vi "Do_ADAM_channel.vi"(3 "Current Time (sec)":dbl, 4 "Scan Period":dbl format="%.2f", 5 "Previous Scan Value":dbl format="%.2f", 6 "Present scan array":dbl[](array[numeric]) format="%.2f", 7 "Value to Output":dbl format="%.2f", 8 "Ch Description":T1 {"Duty" format="%016b"; "D" format="%#_5g"; "C" format="%#_5g"; "B" format="%#_5g"; "A" format="%#_5g"}, 9 "Ch names":string[](array[string])) -> (0 "Scan comment":string, 1 "Output":dbl format="%.3f", 2 "execTime":dbl caption="Execution Time" format="%_3ps")   [LabVIEW 2022 SP3]
uses:
  ADAM Client/Sub VIs/ADAM Controls/Ch_description_ADAM.ctl
  ADAM Client/Sub VIs/ADAM Controls/Module_type_ADAM.ctl
  ADAM Client/Sub VIs/ADAM Controls/Function_ADAM.ctl
  ADAM Client/Sub VIs/ADAM Controls/Channel_State.ctl
  ADAM Client/Sub VIs/ADAM Controls/Calib_type_ADAM.ctl
  ADAM Client/Sub VIs/ADAM Controls/Address.ctl
  ADAM Serial/Instrument drivers/TENMA 72-2xxx PSU/ctls/TENMA 72-2xxx commands.ctl
  ADAM Client/Sub VIs/ADAM Controls/Remember_value_mode.ctl
  ADAM Serial/Instrument drivers/Arduino/ctls_and_globals/Arduino tx msg cluster.ctl
  Anemometry/Anemometry Sub Vis/Controls/In_Range.ctl
  ADAM Client/Sub VIs/ADAM Controls/Update_scan_value.ctl
  Anemometry/Anemometry Sub Vis/Globals/Gas_management_global.vi
  ADAM_Global.vi
  Anemometry/Anemometry Sub Vis/Globals/EnFlo_Tunnel_Global.vi
  Anemometry/Anemometry Sub Vis/Globals/Constants_global.vi
  <vilib>/Analysis/NI_AALBase.lvlib
panel:
  in  "MaxAge(s)":dbl=1.5
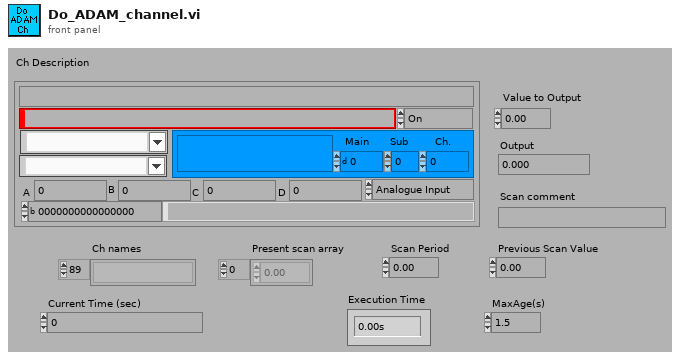
[diagram p1: front panel]
types:
  T1 = typedef "Ch_description_ADAM.ctl" = cluster{"Ch Name":string, "Type":T2, "Function":T3, "Ch State":T4, "Calibration type":T5, "A":dbl, "B":dbl, "C":dbl, "D":dbl, "Comments":string, "Address":T6, "String":string, "Duty":u16}
  T2 = typedef "Module_type_ADAM.ctl" = string
  T3 = typedef "Function_ADAM.ctl" = enum16{"Analogue Input", "Digital Input", "Event counter", "Event rate", "Analogue Output", "Digital Output", "Relay Output"}
  T4 = typedef "Channel_State.ctl" = enum16{"On", "Off", "Always On", "Always Off"}
  T5 = typedef "Calib_type_ADAM.ctl" = string
  T6 = typedef "Address.ctl" = cluster{"Main":i32, "Ch.":i32, "Sub":i32, "Port Name":string}
  T7 = typedef "TENMA 72-2xxx commands.ctl" = string
  T8 = typedef "Remember_value_mode.ctl" = enum16{"Read only", "Read and Write"}
  T9 = typedef "In_Range.ctl" = enum16{"%", "±", "% & ±"}
  T10 = enum16{"Append to Global", "Read Global then Clear"}
  T11 = typedef "Update_scan_value.ctl" = cluster{"Channel Name":string, "New Value":dbl, "!Auto_Off":bool}
  T12 = typedef "Arduino tx msg cluster.ctl" = cluster{"dest":u8, "A/D/C/I":string, "R/W":string, "chan":u8, "val (float)":sgl}
  T13 = typedef "Client_State_Cluster.ctl" = cluster{"Client Name":string, "Traverse level State":T14, "People to Email":string[], "Next Contact Time":dbl}
  T14 = typedef "Traverse_Level_State.ctl" = enum16{"Running", "Complete"}
  T15 = typedef "Modbus error cluster.ctl" = cluster{"Checksum ok":bool, "Modbus exception code":T16, "Response from correct drive":bool, "Comms error":errorcluster}
  T16 = typedef "Exception codes.ctl" = u8
  T17 = typedef "Extended drive status bits.ctl" = cluster{"Ready":bool, "Running":bool, "Tripped":bool, "Standby":bool, "Fire mode":bool, "Reserved (0)":bool, "Speed set-point reached":bool, "Below minimum speed":bool, "Overload":bool, "Mains loss":bool, "Heatsink >85°C":bool, "Control board >80°C":bool, "Switching frequency reduction":bool, "Reverse rotation":bool, "Reserved (0)":bool, "Live toggle bit":bool}
  T18 = typedef "Motor data.ctl" = cluster{"Motor RPM (/min)":dbl, "Motor current (A)":dbl, "Motor power (kW)":dbl, "Motor torque (%)":dbl}
  T19 = typedef "Further motor and drive data.ctl" = cluster{"Motor RMS voltage (V)":dbl, "Drive heatsink temperature (°C)":dbl, "Drive internal temperature (°C)":dbl, "Drive DC bus voltage (V)":dbl, "Drive fault code":T20}
  T20 = typedef "Drive fault codes.ctl" = u8
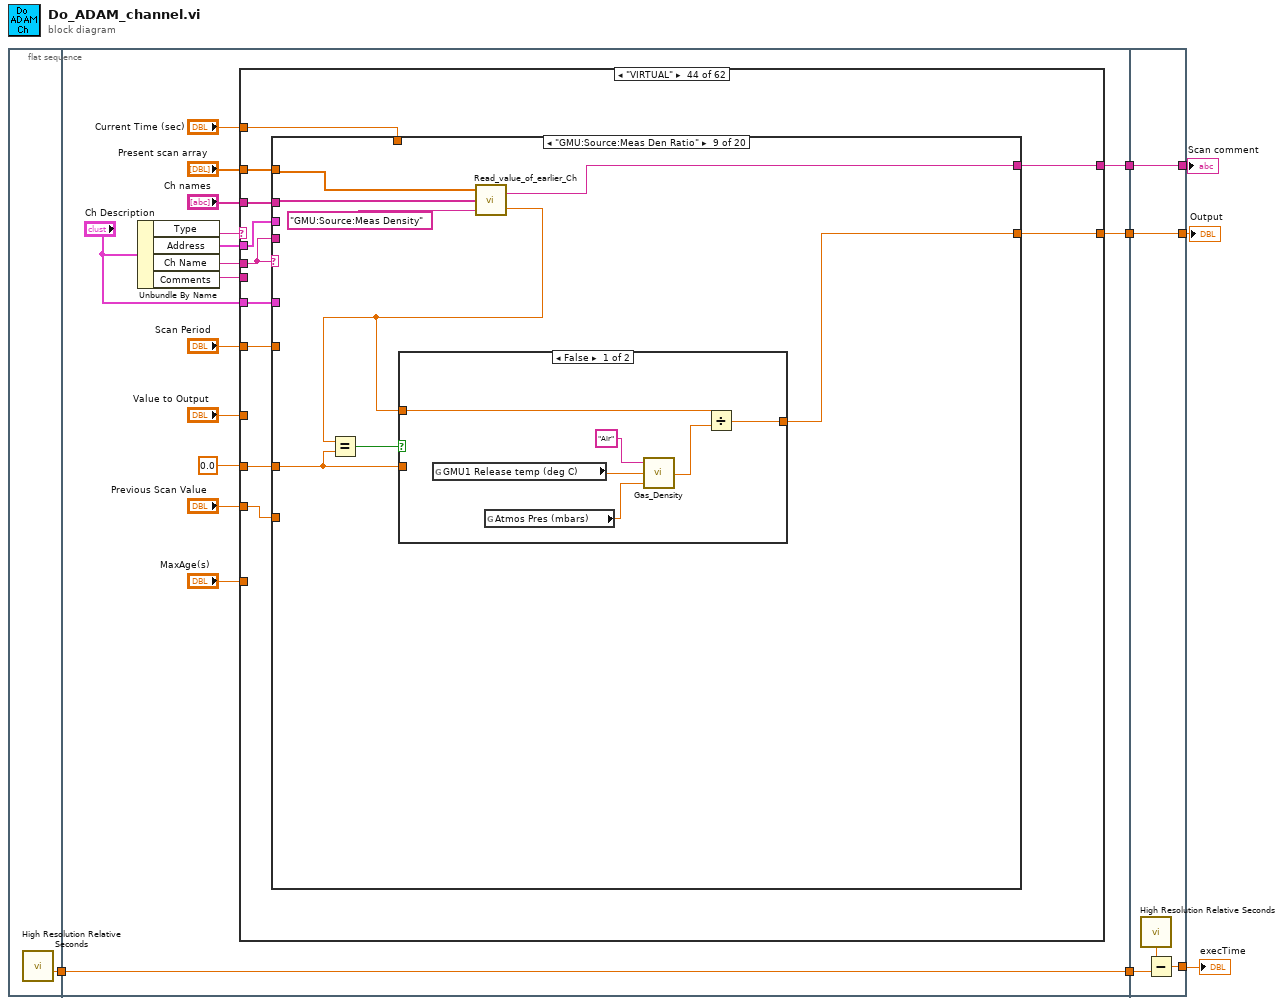
[diagram p0: block diagram]
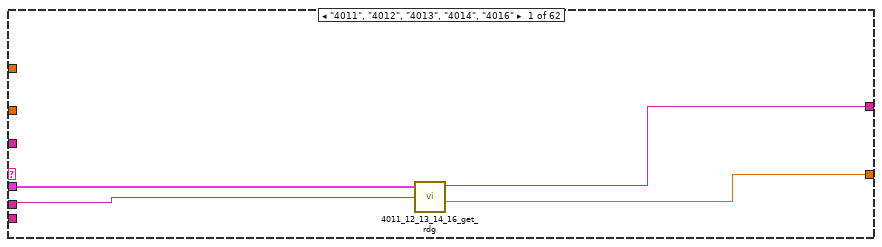
[diagram p2: hidden frame]
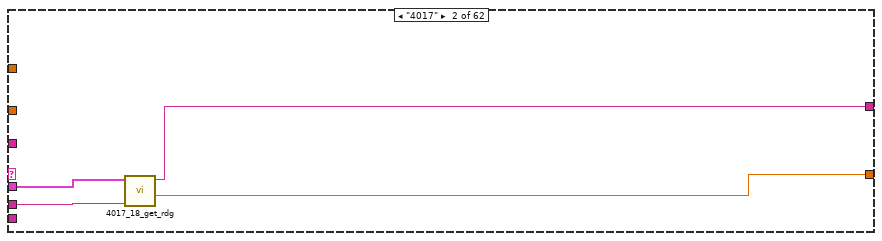
[diagram p3: hidden frame]
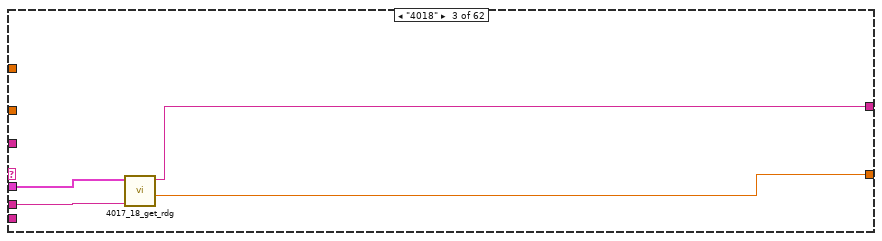
[diagram p4: hidden frame]
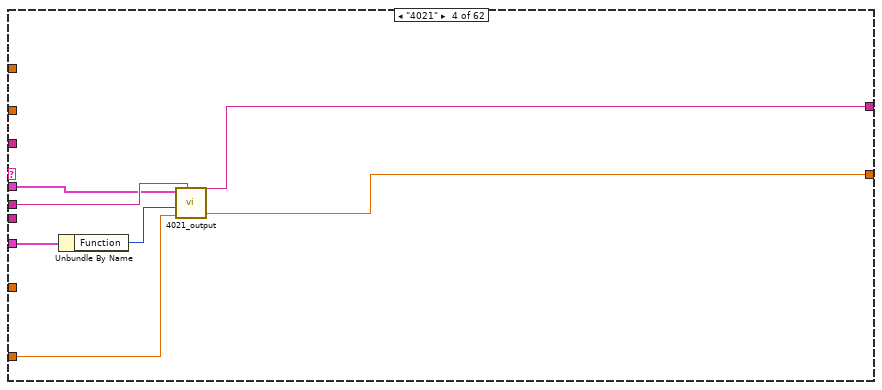
[diagram p5: hidden frame]
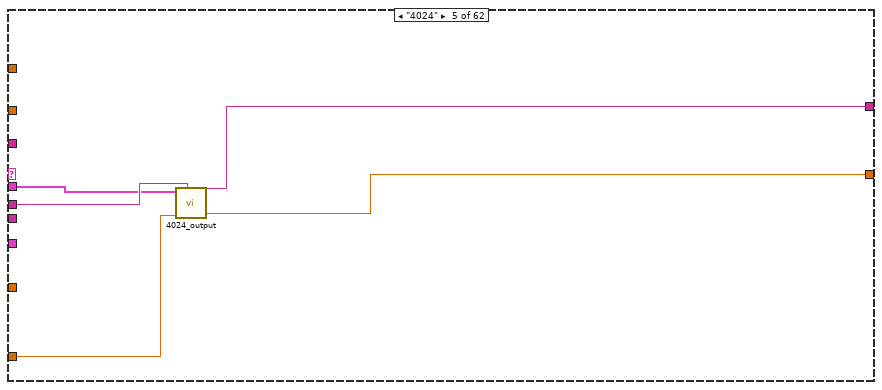
[diagram p6: hidden frame]
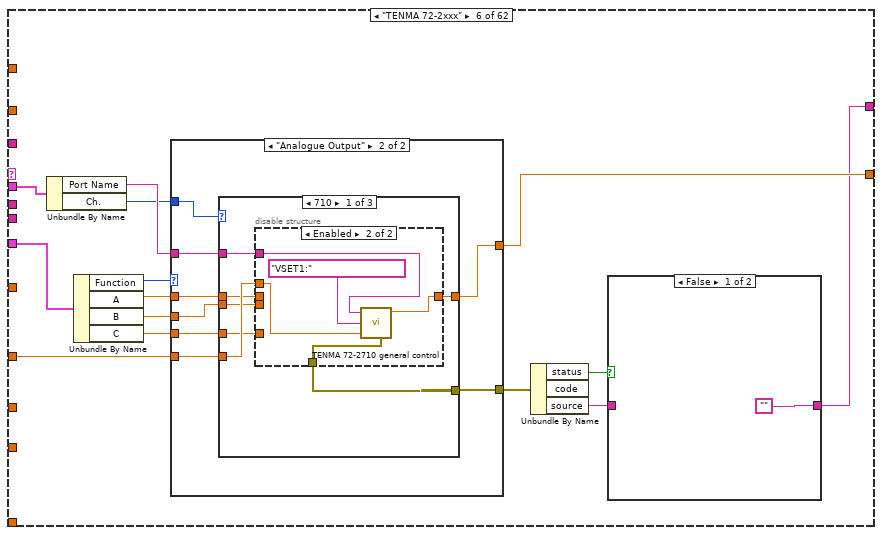
[diagram p7: hidden frame]
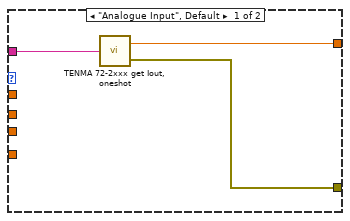
[diagram p8: hidden frame]
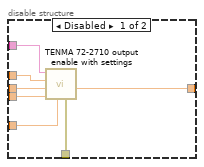
[diagram p9: hidden frame]
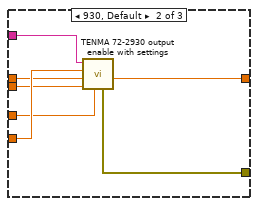
[diagram p10: hidden frame]
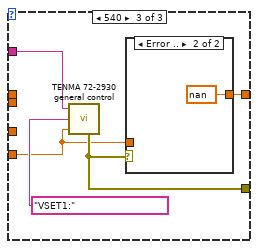
[diagram p11: hidden frame]
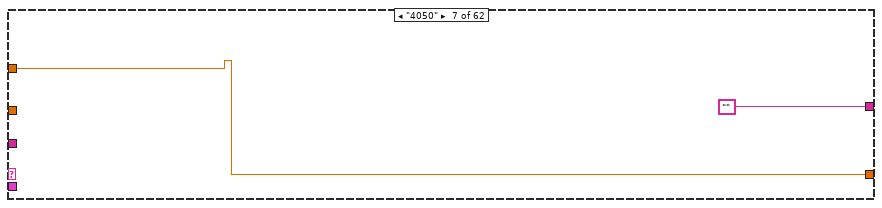
[diagram p14: hidden frame]
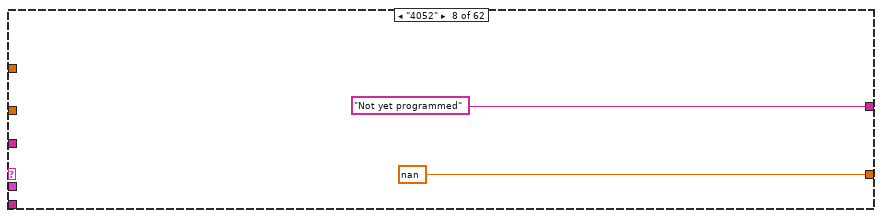
[diagram p15: hidden frame]
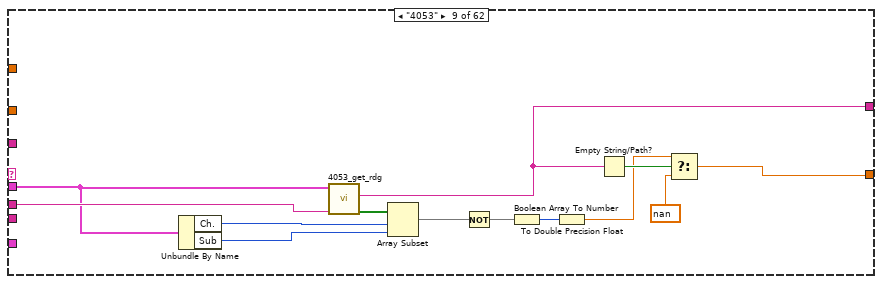
[diagram p16: hidden frame]
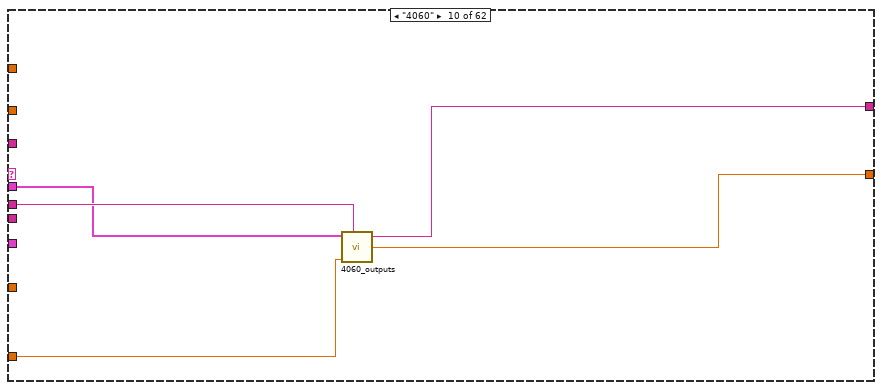
[diagram p17: hidden frame]
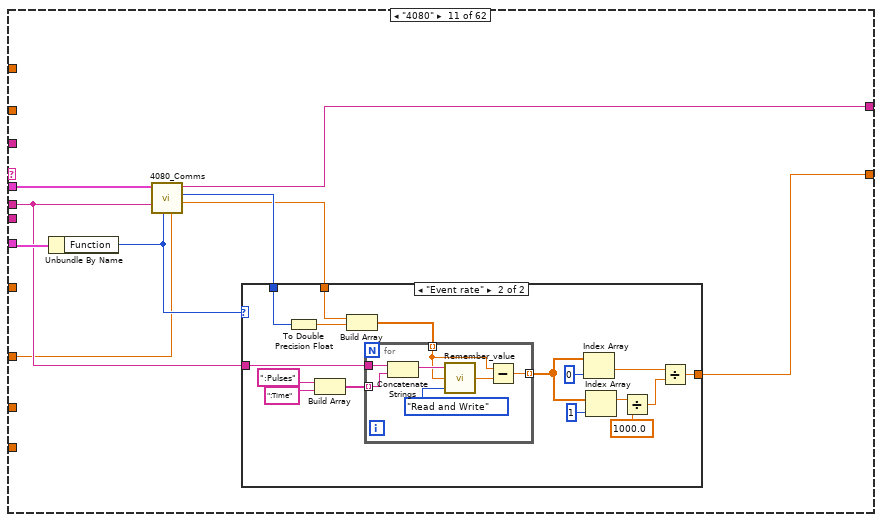
[diagram p18: hidden frame]
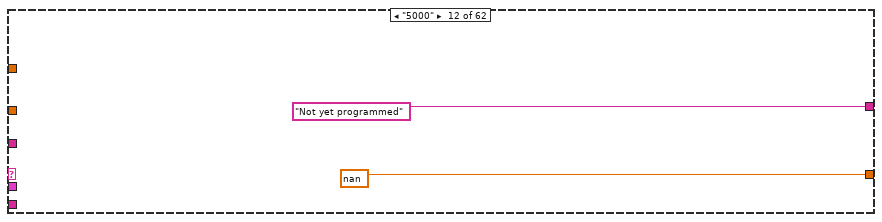
[diagram p20: hidden frame]
diagram:
  n1 = flat-sequence {
    tunnel: [w8] -> w3
    tunnel: [w11] -> w5
    tunnel: [w10] -> w4
    tunnel: w3 -> [w9]
    tunnel: [w9] -> w2
    tunnel: [w1603] -> w6
    tunnel: [w1604] -> w7
    tunnel: w5 -> [w1604]
    tunnel: w4 -> [w1603]
    tunnel: w2 -> [w1601]
    tunnel: [w1600] -> w1
    frame #0 {
      n2 = call <vilib>:"High Resolution Relative Seconds.vi"() -> ("relative seconds"=w8:dbl)
    }
    frame #1 {
      n3 = Unbundle By Name("Ch Description") -> ("Type"=w14:T2, "Address"=w22:T6, "Ch Name"=w16:string, "Comments"=w20:string)
      n4 = case shown="\"VIRTUAL\"" w14 {
        tunnel: [w27 w31 w35 w42 w47 w60 w109 nan w114 w128 w137 nan w167 w177 w209 w217 w238 w260 w280 w297 w313 w330 w360 w381 w486 w604 w606 nan w613 w615 w619 w626 w628 w644 w658 w662 w666 w673 w674 w680 w743 nan w752 w772 w1324 w1334 w1346 w1358 w1372 w1377 w1389 w1396 w1399 w1404 w1410 w1415 w1438 w1460 w1494 w1536 w1592 0.0 ("Output")] -> w10
        tunnel: [w28 w32 w36 w43 w48 w57 "" "Not yet programmed" w117 w129 w139 "Not yet programmed" w168 w180 w210 w216 w239 w261 w279 w296 w316 w332 w355 w380 w485 w605 w607 "Not yet programmed" w612 w616 w620 w625 w629 w643 w657 w663 w667 w672 w678 w682 w744 "Not yet programmed" "" w771 w1325 w1332 "" "" w1371 w1378 w1390 "" w1400 "" w1409 "" "Crazy time based random number!" w1449 w1495 w1537 w1591 "Warning; unmatched case in Do_ADAM_channel" ("Status note")] -> w11
        tunnel: w22 -> [w25 w29 w33 w37 w44 w61 _ _ w118 w127 w131 _ w169 w181 w211 w215 w240 w262 w294 w311 w328 w345 w371 w385 w490 w603 w608 _ _ _ _ w623 w627 w646 _ _ w669 w670 w676 w684 w749 _ w761 w763 _ _ _ _ _ _ _ _ _ _ _ _ _ _ w1499 w1538 _ _]
        tunnel: "Ch Description" -> [_ _ _ w41 _ w55 _ _ _ _ w138 _ _ w170 _ w214 w237 w259 _ _ _ _ _ _ _ _ _ _ w614 w618 w622 _ _ _ w659 w665 _ _ _ w683 _ _ _ w765 w1329 w1338 _ _ w1374 w1380 w1394 _ w1401 w1405 w1411 _ _ _ w1492 _ w1590 _]
        tunnel: w16 -> [w26 w30 w34 w38 w45 _ _ _ w125 w130 w134 _ w166 w176 w208 w212 w234 w256 w278 w295 w312 w329 w347 w377 w482 _ _ _ _ _ _ w624 _ w645 _ _ w668 w671 w677 w681 w748 _ _ w768 _ _ _ w1354 _ _ _ _ _ _ _ _ _ w1456 _ w1531 _ _]
        tunnel: "Ch names" -> [_ _ _ _ _ _ _ _ _ _ _ _ _ _ _ _ _ _ _ _ _ _ _ _ _ _ _ _ _ _ _ _ _ _ _ _ _ _ _ _ _ _ _ w770 w1330 w1337 _ _ w1375 w1381 w1395 _ w1402 _ _ _ _ _ _ _ w1597 _]
        tunnel: "Present scan array" -> [_ _ _ _ _ _ _ _ _ _ _ _ _ _ _ _ _ _ _ _ _ _ _ _ _ _ _ _ _ _ _ _ _ _ _ _ _ _ _ _ _ _ _ w769 w1328 w1335 _ _ w1373 w1379 w1393 _ w1403 _ _ _ _ _ _ _ w1595 _]
        tunnel: w20 -> [_ _ _ _ _ _ _ _ _ _ _ _ _ _ _ _ _ _ _ _ _ _ _ _ _ _ _ _ _ _ _ _ _ _ _ _ _ _ _ _ _ _ _ _ _ _ _ _ _ _ _ _ _ _ _ _ _ _ _ _ _ _]
        tunnel: "Value to Output" -> [_ _ _ w39 w46 w53 _ _ _ w126 w132 _ _ w172 _ w213 w235 w257 _ _ w314 w331 _ _ _ _ _ _ w611 w617 w621 _ _ w642 w660 w664 _ _ _ w679 _ _ w756 _ w1326 _ _ _ _ _ w1391 _ _ _ _ _ _ _ w1488 _ w1596 _]
        tunnel: "Scan Period" -> [_ _ _ _ _ _ _ _ _ _ _ _ _ _ _ _ _ _ _ _ _ _ _ _ _ _ _ _ _ _ _ _ _ _ _ _ _ _ _ _ _ _ _ w767 w1327 w1336 _ _ _ _ w1392 _ _ _ w1407 w1416 _ _ _ _ w1593 _]
        tunnel: "Previous Scan Value" -> [_ _ _ _ _ _ _ _ _ _ _ _ _ _ _ _ _ _ w282 w299 _ _ _ w379 w484 _ _ _ _ _ _ _ _ _ _ _ _ _ _ _ _ _ _ w766 w1323 _ w1346 _ w1370 w1376 w1388 w1396 _ _ w1408 w1413 _ _ _ _ w1594 _]
        tunnel: 0.0 -> [_ _ _ _ _ _ _ _ _ _ _ _ _ _ _ _ _ _ _ _ _ _ _ _ _ _ _ _ _ _ _ _ _ _ _ _ _ _ _ _ _ _ _ w764 _ _ _ _ _ _ _ _ _ _ _ _ _ _ _ _ _ _]
        tunnel: "MaxAge(s)" -> [_ _ _ _ _ _ _ _ _ _ _ _ _ _ _ _ _ _ _ _ _ _ _ _ _ _ _ _ _ _ _ _ _ _ w656 w661 _ _ _ _ _ _ _ _ _ _ _ _ _ _ _ _ _ _ _ _ _ _ _ _ _ _]
        tunnel: "Current Time (sec)" -> [_ _ _ _ _ _ w109 _ _ _ _ _ _ _ _ _ _ _ _ _ _ _ _ _ _ _ _ _ _ _ _ _ _ _ _ _ _ _ _ _ _ _ _ w762 _ _ _ _ _ _ _ _ _ _ _ _ w1431 w1439 _ _ _ _]
        frame "4011", "4012", "4013", "4014", "4016" {
          n5 = call "4011_12_13_14_16_get_rdg.vi"("Address"=w25, "Channel Name"=w26) -> ("Comment"=w28:string, "Reading"=w27:dbl)  [unwired: 1 in, 2 out]
        }
        frame "4017" {
          n6 = call "4017_18_get_rdg.vi"("Channel Name"=w30, "Address"=w29) -> ("Reading"=w31:dbl, "Comment"=w32:string)  [unwired: 2 in, 2 out]
        }
        frame "4018" {
          n7 = call "4017_18_get_rdg.vi"("Channel Name"=w34, "Address"=w33) -> ("Reading"=w35:dbl, "Comment"=w36:string)  [unwired: 2 in, 2 out]
        }
        frame "4021" {
          n8 = Unbundle By Name(w41) -> ("Function"=w40:T3)
          n9 = call "4021_output.vi"("Address"=w37, "Function"=w40, "Set to:"=w39, "Channel Name"=w38) -> ("Comment"=w43:string, "Reading"=w42:dbl)  [unwired: 1 in, 1 out]
        }
        frame "4024" {
          n10 = call "4024_output.vi"("Address"=w44, "Set to:"=w46, "Channel Name"=w45) -> ("Comment"=w48:string, "Reading"=w47:dbl)  [unwired: 3 in]
        }
        frame "TENMA 72-2xxx" {
          n11 = Unbundle By Name(w61) -> ("Port Name"=w62:string, "Ch."=w49:i32)
          n12 = Unbundle By Name(w55) -> ("Function"=w54:T3, "A"=w52:dbl, "B"=w51:dbl, "C"=w50:dbl)
          n13 = case shown="\"Analogue Output\"" w54 {
            tunnel: w62 -> [w65 w73]
            tunnel: [w64 w67] -> w60
            tunnel: [w63 w68] -> w59
            tunnel: w53 -> [_ w72]
            tunnel: w52 -> [_ w71]
            tunnel: w51 -> [_ w70]
            tunnel: w50 -> [_ w69]
            tunnel: w49 -> [_ w66]
            frame "Analogue Input", Default {
              n14 = call "TENMA 72-2xxx get Iout, oneshot.vi"("Port"=w65) -> ("Iout (A)"=w64:sgl, "error out"=w63:errorcluster)
            }
            frame "Analogue Output" {
              n15 = case shown="710" w66 {
                tunnel: w73 -> [w80 w99 w104]
                tunnel: w72 -> [w79 w98 w100]
                tunnel: w71 -> [w78 w97 _]
                tunnel: w70 -> [w77 w96 _]
                tunnel: w69 -> [w76 w95 _]
                tunnel: [w75 w94 w102] -> w68
                tunnel: [w74 w93 w101] -> w67
                frame 710 {
                  n16 = disable-structure shown="Enabled" {
                    disable-tunnel: w80 -> [w87 w91]
                    disable-tunnel: w79 -> [w86 w88]
                    disable-tunnel: w78 -> [w85 _]
                    disable-tunnel: w77 -> [w84 _]
                    disable-tunnel: w76 -> [w83 _]
                    disable-tunnel: [w82 w89] -> w75
                    disable-tunnel: [w81 w90] -> w74
                    frame Disabled {
                      n17 = call "TENMA 72-2710 output enable with settings.vi"("Initial wait (ms)"=w83, "Running current limit (A)"=w84, "Initial current limit (A)"=w85, "Voltate output (V)"=w86, "Port"=w87) -> ("Returned voltage output (V)"=w81:sgl, "Error out"=w82:errorcluster)  [unwired: 2 in, 3 out]
                    }
                    frame Enabled {
                      n18 = call "TENMA 72-2710 general control.vi"("Value to set"=w88, "Command"=T7 "VSET1:", "Port"=w91) -> ("error out"=w89:errorcluster, "Returned value"=w90:sgl)  [unwired: 1 in, 3 out]
                    }
                  }
                }
                frame 930, Default {
                  n19 = call "TENMA 72-2930 output enable with settings.vi"("Initial wait (ms)"=w95, "Running current limit (A)"=w96, "Initial current limit (A)"=w97, "Voltate output (V)"=w98, "Port"=w99) -> ("Returned voltage output (V)"=w93:sgl, "Error out"=w94:errorcluster)  [unwired: 2 in, 3 out]
                }
                frame 540 {
                  n20 = call "TENMA 72-2930 general control.vi"("Value to set"=w100, "Command"=T7 "VSET1:", "Port"=w104) -> ("error out"=w102:errorcluster)  [unwired: 1 in, 4 out]
                  n21 = case shown="Error .." w102 {
                    tunnel: [w105 nan ("Value to Output")] -> w101
                    tunnel: w100 -> [w105 _]
                    frame No Error {
                    }
                    frame Error {
                    }
                  }
                }
              }
            }
          }
          n22 = Unbundle By Name(w59) -> ("status"=w58:bool, "source"=w56:string)  [unwired: 1 out]
          n23 = case shown="False" w58 {
            tunnel: ["" w108] -> w57
            tunnel: w56 -> [_ w108]
            frame False {
            }
            frame True {
            }
          }
        }
        frame "4050" {
        }
        frame "4052" {
        }
        frame "4053" {
          n24 = Unbundle By Name(w118) -> ("Ch."=w119:i32, "Sub"=w124:i32)
          n25 = call "4053_get_rdg.vi"("Channel Name"=w125, "Address"=w118) -> ("Boolean array"=w123:bool[], "Comment"=w117:string)  [unwired: 2 in, 2 out]
          n26 = Array Subset(array=w123, index=w119, length=w124) -> (w122:bool[])
          n27 = Not(x=w122) -> (.not. x?=w120:bool[])
          n28 = Boolean Array To Number(Boolean array=w120) -> (number=w121:u32)
          n29 = To Double Precision Float(number=w121) -> (double precision float=w115:dbl)
          n30 = Empty String/Path?(string/path=w117) -> (empty?=w116:bool)
          n31 = Select(t=w115, s=w116, f=nan) -> (s? t:f=w114:dbl)
        }
        frame "4060" {
          n32 = call "4060_outputs.vi"("Address"=w127, "Value to Output"=w126, "Channel Name"=w130) -> ("Comment"=w129:string, "Reading"=w128:dbl)  [unwired: 2 in, 1 out]
        }
        frame "4080" {
          n33 = Unbundle By Name(w138) -> ("Function"=w133:T3)
          n34 = call "4080_Comms.vi"("Value to display"=w132, "Function"=w133, "Channel Name"=w134, "Address"=w131) -> ("Reading"=w135:dbl, "millisecond timer value"=w136:u32, "Comment"=w139:string)  [unwired: 2 in, 1 out]
          n35 = case shown="\"Event rate\"" w133 {
            tunnel: w134 -> [_ w156]
            tunnel: w136 -> [_ w149]
            tunnel: [w140 w141] -> w137
            tunnel: w135 -> [w140 w150]
            frame "Event counter", Default {
            }
            frame "Event rate" {
              n36 = To Double Precision Float(number=w149) -> (double precision float=w148:dbl)
              n37 = Build Array(":Pulses", ":Time") -> (w151:string[])
              n38 = Build Array(w150, w148) -> (w147:dbl[])
              n39 = for {
                tunnel: w156 -> [w160]
                tunnel: [w161] -> w144 mode=indexing
                tunnel: w151 -> [w158] mode=indexing
                tunnel: w147 -> [w157] mode=indexing
                n40 = Concatenate Strings(w160, w158) -> (w159:string)
                n41 = call "Remember_value.vi"("Mode"=Remember_value_mode."Read and Write", "Input Value"=w157, "Ch name"=w159) -> ("Output Value"=w162:dbl)
                n42 = Subtract(x=w157, y=w162) -> (x-y=w161:dbl)
              }
              n43 = Index Array(array=w144, index=0) -> (element=w142:dbl)
              n44 = Index Array(array=w144, index=1) -> (element=w143:dbl)
              n45 = Divide(x=w143, y=1000.0) -> (x/y=w154:dbl)
              n46 = Divide(x=w142, y=w154) -> (x/y=w141:dbl)
            }
          }
        }
        frame "5000" {
        }
        frame "5017", "5018" {
          n47 = call "5017_18_get_rdg.vi"("Address (all reqd.)"=w169, "Channel Name"=w166) -> ("Comment"=w168:string, "Reading"=w167:dbl)  [unwired: 3 out]
        }
        frame "5024" {
          n48 = Less Than 0?(x=w172) -> (x < 0?=w175:bool)
          n49 = Unbundle By Name(w170) -> ("Calibration type"=w171:T5)
          n50 = case shown="False" w175 {
            tunnel: [w187 0.0 ("t")] -> w173
            tunnel: w172 -> [w185 _]
            tunnel: w171 -> [w186 _]
            tunnel: w170 -> [w184 _]
            frame False {
              n51 = case shown="\"Dx^3 + Cx^2 + Bx + A\"" w186 {
                tunnel: w185 -> [w188 w191 w197 w203]
                tunnel: w184 -> [_ w194 w200 w206]
                tunnel: [w188 w189 w195 w201] -> w187
                frame "Raw", Default {
                }
                frame "Bx + A" {
                  n52 = Unbundle By Name(w194) -> ("A"=w193:dbl)
                  n53 = Equal?(x=w193, y=w191) -> (x = y?=w192:bool)
                  n54 = Select(t=0.0, s=w192, f=w191) -> (s? t:f=w189:dbl)
                }
                frame "Cx^2 + Bx + A" {
                  n55 = Unbundle By Name(w200) -> ("A"=w199:dbl)
                  n56 = Equal?(x=w199, y=w197) -> (x = y?=w198:bool)
                  n57 = Select(t=0.0, s=w198, f=w197) -> (s? t:f=w195:dbl)
                }
                frame "Dx^3 + Cx^2 + Bx + A" {
                  n58 = Unbundle By Name(w206) -> ("A"=w205:dbl)
                  n59 = Equal?(x=w205, y=w203) -> (x = y?=w204:bool)
                  n60 = Select(t=0.0, s=w204, f=w203) -> (s? t:f=w201:dbl)
                }
              }
            }
            frame True {
            }
          }
          n61 = call "5024_set_output.vi"("Set to:"=w173, "Address (all reqd.)"=w181, "Channel Name"=w176) -> ("Comment"=w180:string, "Good Reply"=w178:bool)  [unwired: 2 out]
          n62 = case shown="\"Bx + A\", Default" w171 {
            tunnel: [w182 w183] -> w174
            tunnel: w173 -> [w182 _]
            tunnel: w172 -> [_ w183]
            frame "Raw" {
            }
            frame "Bx + A", Default {
            }
          }
          n63 = Select(t=w174, s=w178, f=nan) -> (s? t:f=w177:dbl)
        }
        frame "5051" {
          n64 = call "5051_56_get_inputs.vi"("Address (Main, Sub reqd.)"=w211, "Channel Name"=w208) -> ("Comment"=w210:string, "Single output"=w209:dbl)  [unwired: 3 out]
        }
        frame "5056" {
          n65 = Unbundle By Name(w214) -> ("Function"=w218:T3)
          n66 = case shown="\"Relay Output\"" w218 {
            tunnel: w215 -> [_ w224 w233]
            tunnel: ["This function is not available" w225 w231] -> w216
            tunnel: [nan ("A") w222 w228] -> w217
            tunnel: w213 -> [_ _ w227]
            tunnel: w212 -> [_ w221 w226]
            frame "Analogue Input", Default {
            }
            frame "Digital Input" {
              # "Readback value"
              n67 = call "5060_check_outputs.vi"("Address (Main, Sub reqd.)"=w224, "Channel Name"=w221) -> ("Comment"=w225:string, "Single Channel"=w223:i16)  [unwired: 3 out]
              n68 = To Double Precision Float(number=w223) -> (double precision float=w222:dbl)
            }
            frame "Relay Output" {
              # "Sets single o/p channel"
              n69 = Greater Than 0?(x=w227) -> (x > 0?=w232:bool)
              n70 = call "5056_60_set_single_output.vi"("Channel Name"=w226, "Address (all reqd.)"=w233, "Set state:"=w232) -> ("Comment"=w231:string, "Good Reply"=w230:bool)  [unwired: 2 out]
              n71 = Select(t=w227, s=w230, f=nan) -> (s? t:f=w228:dbl)
            }
          }
        }
        frame "5060" {
          n72 = Unbundle By Name(w237) -> ("Function"=w236:T3)
          n73 = case shown="\"Relay Output\"" w236 {
            tunnel: w240 -> [_ w246 w255]
            tunnel: ["This function is not available" w247 w253] -> w239
            tunnel: [nan ("A") w244 w250] -> w238
            tunnel: w235 -> [_ _ w249]
            tunnel: w234 -> [_ w243 w248]
            frame "Analogue Input", Default {
            }
            frame "Digital Input" {
              # "Readback value"
              n74 = call "5060_check_outputs.vi"("Address (Main, Sub reqd.)"=w246, "Channel Name"=w243) -> ("Comment"=w247:string, "Single Channel"=w245:i16)  [unwired: 3 out]
              n75 = To Double Precision Float(number=w245) -> (double precision float=w244:dbl)
            }
            frame "Relay Output" {
              # "Sets single o/p channel"
              n76 = Greater Than 0?(x=w249) -> (x > 0?=w254:bool)
              n77 = call "5056_60_set_single_output.vi"("Channel Name"=w248, "Address (all reqd.)"=w255, "Set state:"=w254) -> ("Comment"=w253:string, "Good Reply"=w252:bool)  [unwired: 2 out]
              n78 = Select(t=w249, s=w252, f=nan) -> (s? t:f=w250:dbl)
            }
          }
        }
        frame "6060" {
          n79 = Unbundle By Name(w259) -> ("Function"=w258:T3)
          n80 = case shown="\"Relay Output\"" w258 {
            tunnel: w262 -> [_ w268 w277]
            tunnel: ["This function is not available" w269 w275] -> w261
            tunnel: [nan ("A") w266 w272] -> w260
            tunnel: w257 -> [_ _ w271]
            tunnel: w256 -> [_ w265 w270]
            frame "Analogue Input", Default {
            }
            frame "Digital Input" {
              n81 = call "6060_read_all_I-O.vi"("Address (Main, Sub reqd.)"=w268, "Channel Name"=w265) -> ("Comment"=w269:string, "Single Input Channel"=w267:i16)  [unwired: 3 out]
              n82 = To Double Precision Float(number=w267) -> (double precision float=w266:dbl)
            }
            frame "Relay Output" {
              # "Sets single o/p channel"
              n83 = Greater Than 0?(x=w271) -> (x > 0?=w276:bool)
              n84 = call "6060_set_single_output.vi"("Channel Name"=w270, "Address (Main, Ch requd.)"=w277, "Set state:"=w276) -> ("Comment"=w275:string, "Good Reply"=w274:bool)  [unwired: 2 out]
              n85 = Select(t=w271, s=w274, f=nan) -> (s? t:f=w272:dbl)
            }
          }
        }
        frame "Arduino A_in" {
          w288 = T12 {"dest"=1, "A/D/C/I"="A", "R/W"="R", "chan"=1, "val (float)"=0.0}  # Tx msg cluster
          # "Analogue read case"
          n86 = Unbundle By Name(w294) -> ("Port Name"=w285:string, "Main"=w286:i32, "Ch."=w287:i32)
          n87 = To Unsigned Byte Integer(number=w286) -> (unsigned 8bit integer=w293:u8)
          n88 = To Unsigned Byte Integer(number=w287) -> (unsigned 8bit integer=w291:u8)
          n89 = Bundle By Name(cluster=w288, "dest"=w293, "A/D/C/I"="A" ("A/D"), "R/W"="R", "chan"=w291, "val (float)"=sgl 0.0) -> (w284:T12)
          n90 = call "Arduino generic wrapper.vi"("Tx msg cluster"=w284, "Channel Name"=w278, "Port name"=w285) -> ("Scan comment"=w279:string, "Output"=w281:dbl)
          n91 = Empty String/Path?(string/path=w279) -> (empty?=w283:bool)
          n92 = Select(t=w281, s=w283, f=w282) -> (s? t:f=w280:dbl)
        }
        frame "Pref" {
          w305 = T12 {"dest"=1, "A/D/C/I"="A", "R/W"="R", "chan"=1, "val (float)"=0.0}  # Tx msg cluster
          # "Analogue read case"
          n93 = Unbundle By Name(w311) -> ("Port Name"=w302:string, "Main"=w303:i32, "Ch."=w304:i32)
          n94 = To Unsigned Byte Integer(number=w303) -> (unsigned 8bit integer=w310:u8)
          n95 = To Unsigned Byte Integer(number=w304) -> (unsigned 8bit integer=w308:u8)
          n96 = Bundle By Name(cluster=w305, "dest"=w310, "A/D/C/I"="P" ("A/D"), "R/W"="R", "chan"=w308, "val (float)"=sgl 0.0) -> (w301:T12)
          n97 = call "Arduino generic wrapper.vi"("Tx msg cluster"=w301, "Channel Name"=w295, "Port name"=w302) -> ("Scan comment"=w296:string, "Output"=w298:dbl)
          n98 = Empty String/Path?(string/path=w296) -> (empty?=w300:bool)
          n99 = Select(t=w298, s=w300, f=w299) -> (s? t:f=w297:dbl)
        }
        frame "Arduino A_out" {
          w323 = T12 {"dest"=1, "A/D/C/I"="A", "R/W"="R", "chan"=1, "val (float)"=0.0}  # Tx msg cluster
          # "Analogue write case"
          n100 = Unbundle By Name(w328) -> ("Port Name"=w320:string, "Main"=w321:i32, "Ch."=w322:i32)
          n101 = To Unsigned Byte Integer(number=w321) -> (unsigned 8bit integer=w327:u8)
          n102 = To Unsigned Byte Integer(number=w322) -> (unsigned 8bit integer=w326:u8)
          n103 = To Single Precision Float(number=w314) -> (single precision float=w318:sgl)
          n104 = Bundle By Name(cluster=w323, "dest"=w327, "A/D/C/I"="A" ("A/D"), "R/W"="W", "chan"=w326, "val (float)"=w318) -> (w319:T12)
          n105 = call "Arduino generic wrapper.vi"("Tx msg cluster"=w319, "Channel Name"=w312, "Port name"=w320) -> ("Scan comment"=w316:string)  [unwired: 1 out]
          n106 = Empty String/Path?(string/path=w316) -> (empty?=w315:bool)
          n107 = Select(t=w314, s=w315, f=nan ("Reading")) -> (s? t:f=w313:dbl)
        }
        frame "Arduino D_out" {
          w340 = T12 {"dest"=1, "A/D/C/I"="A", "R/W"="R", "chan"=1, "val (float)"=0.0}  # Tx msg cluster
          # "Digital write case"
          n108 = Unbundle By Name(w345) -> ("Port Name"=w337:string, "Main"=w338:i32, "Ch."=w339:i32)
          n109 = To Unsigned Byte Integer(number=w338) -> (unsigned 8bit integer=w344:u8)
          n110 = To Unsigned Byte Integer(number=w339) -> (unsigned 8bit integer=w343:u8)
          n111 = To Single Precision Float(number=w331) -> (single precision float=w335:sgl)
          n112 = Bundle By Name(cluster=w340, "dest"=w344, "A/D/C/I"="D" ("A/D"), "R/W"="W", "chan"=w343, "val (float)"=w335) -> (w336:T12)
          n113 = call "Arduino generic wrapper.vi"("Tx msg cluster"=w336, "Channel Name"=w329, "Port name"=w337) -> ("Scan comment"=w332:string)  [unwired: 1 out]
          n114 = Empty String/Path?(string/path=w332) -> (empty?=w333:bool)
          n115 = Select(t=w331, s=w333, f=nan ("Reading")) -> (s? t:f=w330:dbl)
        }
        frame "Arduino Thermistor" {
          w365 = T12 {"dest"=1, "A/D/C/I"="A", "R/W"="R", "chan"=1, "val (float)"=0.0}  # Tx msg cluster
          # "Thermistor read case"
          # "values not expected in 'normal' operating conditions"
          n116 = Unbundle By Name(w371) -> ("Port Name"=w362:string, "Main"=w363:i32, "Ch."=w364:i32)
          n117 = To Unsigned Byte Integer(number=w363) -> (unsigned 8bit integer=w370:u8)
          n118 = To Unsigned Byte Integer(number=w364) -> (unsigned 8bit integer=w368:u8)
          n119 = Bundle By Name(cluster=w365, "dest"=w370, "A/D/C/I"="A" ("A/D"), "R/W"="R", "chan"=w368, "val (float)"=sgl 0.0) -> (w361:T12)
          n120 = call "Arduino generic wrapper.vi"("Tx msg cluster"=w361, "Channel Name"=w347, "Port name"=w362) -> ("Scan comment"=w351:string, "Output"=w349:dbl)
          n121 = Empty String/Path?(string/path=w351) -> (empty?=w350:bool)
          n122 = Select(t=w349, s=w350, f=nan) -> (s? t:f=w348:dbl)
          n123 = Less?(x=w349, y=-40.0) -> (x < y?=w352:bool)
          n124 = Greater?(x=w349, y=140.0) -> (0:w353:bool)
          n125 = case shown="False" w352 {
            tunnel: [w373 "Faulty thermistor open-circuit;"] -> w354
            tunnel: w353 -> [w372 _]
            frame False {
              n126 = case shown="False" w372 {
                tunnel: ["" "Faulty thermistor short-circuit;"] -> w373
                frame False {
                }
                frame True {
                }
              }
            }
            frame True {
            }
          }
          n127 = Or(x=w352, y=w353) -> (x .or. y?=w357:bool)
          n128 = Select(t=nan ("f"), s=w357, f=w348) -> (s? t:f=w360:dbl)
          n129 = Concatenate Strings(w351, w354) -> (w355:string)
        }
        frame "NaMCU" {
          # "See \"Default\" tab for channel matrix"
          # "PN's \"NaMCU\" devices. Low range pressure transducer with on-board correction, environmental sensor, 2x thermistors, Ain + Aout (5V), Din + Dout"
          n130 = Unbundle By Name(w385) -> ("Port Name"=w382:string, "Main"=w383:i32, "Sub"=w378:i32, "Ch."=w384:i32)
          n131 = case shown="4" w378 {
            tunnel: w384 -> [w395 w420 w441 w457 w473 _]
            tunnel: w383 -> [w394 w419 w440 w456 w472 _]
            tunnel: w382 -> [w393 w418 w439 w455 w471 _]
            tunnel: [w387 w416 w433 w449 w465 0.0 ("Output")] -> w381
            tunnel: [w388 w411 w435 w451 w467 "Warning; invalid Sub being addressed on a NaMCU device in Do_ADAM_channel.vi"] -> w380
            tunnel: w379 -> [w389 w403 w436 w452 w468 _]
            tunnel: w377 -> [w386 w402 w432 w448 w464 _]
            frame 0 {
              w396 = T12 {"dest"=1, "A/D/C/I"="A", "R/W"="R", "chan"=1, "val (float)"=0.0}  # Tx msg cluster
              # "Get pressure (Pa)"
              n132 = To Unsigned Byte Integer(number=w394) -> (unsigned 8bit integer=w401:u8)
              n133 = To Unsigned Byte Integer(number=w395) -> (unsigned 8bit integer=w399:u8)
              n134 = Bundle By Name(cluster=w396, "dest"=w401, "A/D/C/I"="P" ("A/D"), "R/W"="R", "chan"=w399, "val (float)"=sgl 0.0) -> (w392:T12)
              n135 = call "Arduino generic wrapper.vi"("Tx msg cluster"=w392, "Channel Name"=w386, "Port name"=w393) -> ("Scan comment"=w388:string, "Output"=w390:dbl)
              n136 = Empty String/Path?(string/path=w388) -> (empty?=w391:bool)
              n137 = Select(t=w390, s=w391, f=w389) -> (s? t:f=w387:dbl)
            }
            frame 1 {
              w421 = T12 {"dest"=1, "A/D/C/I"="A", "R/W"="R", "chan"=1, "val (float)"=0.0}  # Tx msg cluster
              # "values not expected in 'normal' operating conditions"
              # "Get temperature (deg C)"
              n138 = To Unsigned Byte Integer(number=w419) -> (unsigned 8bit integer=w426:u8)
              n139 = To Unsigned Byte Integer(number=w420) -> (unsigned 8bit integer=w424:u8)
              n140 = Bundle By Name(cluster=w421, "dest"=w426, "A/D/C/I"="T" ("A/D"), "R/W"="R", "chan"=w424, "val (float)"=sgl 0.0) -> (w417:T12)
              n141 = call "Arduino generic wrapper.vi"("Tx msg cluster"=w417, "Channel Name"=w402, "Port name"=w418) -> ("Scan comment"=w407:string, "Output"=w405:dbl)
              n142 = Empty String/Path?(string/path=w407) -> (empty?=w406:bool)
              n143 = Select(t=w405, s=w406, f=w403) -> (s? t:f=w404:dbl)
              n144 = Less?(x=w405, y=-40.0) -> (x < y?=w408:bool)
              n145 = Greater?(x=w405, y=140.0) -> (0:w409:bool)
              n146 = case shown="False" w408 {
                tunnel: [w428 "Faulty thermistor open-circuit;"] -> w410
                tunnel: w409 -> [w427 _]
                frame False {
                  n147 = case shown="True" w427 {
                    tunnel: ["" "Faulty thermistor short-circuit;"] -> w428
                    frame False {
                    }
                    frame True {
                    }
                  }
                }
                frame True {
                }
              }
              n148 = Or(x=w408, y=w409) -> (x .or. y?=w413:bool)
              n149 = Select(t=nan ("f"), s=w413, f=w404) -> (s? t:f=w416:dbl)
              n150 = Concatenate Strings(w407, w410) -> (w411:string)
            }
            frame 2 {
              w442 = T12 {"dest"=1, "A/D/C/I"="A", "R/W"="R", "chan"=1, "val (float)"=0.0}  # Tx msg cluster
              # "Get relative humidity (%)"
              n151 = To Unsigned Byte Integer(number=w440) -> (unsigned 8bit integer=w447:u8)
              n152 = To Unsigned Byte Integer(number=w441) -> (unsigned 8bit integer=w445:u8)
              n153 = Bundle By Name(cluster=w442, "dest"=w447, "A/D/C/I"="H" ("A/D"), "R/W"="R", "chan"=w445, "val (float)"=sgl 0.0) -> (w438:T12)
              n154 = call "Arduino generic wrapper.vi"("Tx msg cluster"=w438, "Channel Name"=w432, "Port name"=w439) -> ("Scan comment"=w435:string, "Output"=w434:dbl)
              n155 = Empty String/Path?(string/path=w435) -> (empty?=w437:bool)
              n156 = Select(t=w434, s=w437, f=w436) -> (s? t:f=w433:dbl)
            }
            frame 3 {
              w458 = T12 {"dest"=1, "A/D/C/I"="A", "R/W"="R", "chan"=1, "val (float)"=0.0}  # Tx msg cluster
              # "Get fluid density (kg/m^3)"
              n157 = To Unsigned Byte Integer(number=w456) -> (unsigned 8bit integer=w463:u8)
              n158 = To Unsigned Byte Integer(number=w457) -> (unsigned 8bit integer=w461:u8)
              n159 = Bundle By Name(cluster=w458, "dest"=w463, "A/D/C/I"="R" ("A/D"), "R/W"="R", "chan"=w461, "val (float)"=sgl 0.0) -> (w454:T12)
              n160 = call "Arduino generic wrapper.vi"("Tx msg cluster"=w454, "Channel Name"=w448, "Port name"=w455) -> ("Scan comment"=w451:string, "Output"=w450:dbl)
              n161 = Empty String/Path?(string/path=w451) -> (empty?=w453:bool)
              n162 = Select(t=w450, s=w453, f=w452) -> (s? t:f=w449:dbl)
            }
            frame 4 {
              w474 = T12 {"dest"=1, "A/D/C/I"="A", "R/W"="R", "chan"=1, "val (float)"=0.0}  # Tx msg cluster
              # "Get flow speed (pitot-static equivalent) (m/s)"
              n163 = To Unsigned Byte Integer(number=w472) -> (unsigned 8bit integer=w479:u8)
              n164 = To Unsigned Byte Integer(number=w473) -> (unsigned 8bit integer=w477:u8)
              n165 = Bundle By Name(cluster=w474, "dest"=w479, "A/D/C/I"="U" ("A/D"), "R/W"="R", "chan"=w477, "val (float)"=sgl 0.0) -> (w470:T12)
              n166 = call "Arduino generic wrapper.vi"("Tx msg cluster"=w470, "Channel Name"=w464, "Port name"=w471) -> ("Scan comment"=w467:string, "Output"=w466:dbl)
              n167 = Empty String/Path?(string/path=w467) -> (empty?=w469:bool)
              n168 = Select(t=w466, s=w469, f=w468) -> (s? t:f=w465:dbl)
            }
            frame Default {
              # "dP_sensor and flow speed are time-averaged between calls"
              # "Oh dear, user has created a server channel with an invalid \"sub\" address"
            }
          }
        }
        frame "NaCTA" {
          # "See \"Default\" tab for channel matrix"
          # "PN's \"NaCTA\" devices. Thermistor CTA with on-board calibration drift compensation, environmental sensor, 6-axis IMU."
          n169 = Unbundle By Name(w490) -> ("Port Name"=w487:string, "Main"=w488:i32, "Sub"=w483:i32, "Ch."=w489:i32)
          n170 = case shown="5" w483 {
            tunnel: w489 -> [w500 w525 w546 w562 w578 w594 _]
            tunnel: w488 -> [w499 w524 w545 w561 w577 w593 _]
            tunnel: w487 -> [w498 w523 w544 w560 w576 w592 _]
            tunnel: [w492 w521 w538 w554 w570 w586 0.0 ("Output")] -> w486
            tunnel: [w493 w516 w540 w556 w572 w588 "Warning; invalid Sub being addressed on a NaCTA device in Do_ADAM_channel.vi"] -> w485
            tunnel: w484 -> [w494 w508 w541 w557 w573 w589 _]
            tunnel: w482 -> [w491 w507 w537 w553 w569 w585 _]
            frame 0 {
              w501 = T12 {"dest"=1, "A/D/C/I"="A", "R/W"="R", "chan"=1, "val (float)"=0.0}  # Tx msg cluster
              # "Get atmospheric pressure (Pa)"
              n171 = To Unsigned Byte Integer(number=w499) -> (unsigned 8bit integer=w506:u8)
              n172 = To Unsigned Byte Integer(number=w500) -> (unsigned 8bit integer=w504:u8)
              n173 = Bundle By Name(cluster=w501, "dest"=w506, "A/D/C/I"="P" ("A/D"), "R/W"="R", "chan"=w504, "val (float)"=sgl 0.0) -> (w497:T12)
              n174 = call "Arduino generic wrapper.vi"("Tx msg cluster"=w497, "Channel Name"=w491, "Port name"=w498) -> ("Scan comment"=w493:string, "Output"=w495:dbl)
              n175 = Empty String/Path?(string/path=w493) -> (empty?=w496:bool)
              n176 = Select(t=w495, s=w496, f=w494) -> (s? t:f=w492:dbl)
            }
            frame 1 {
              w526 = T12 {"dest"=1, "A/D/C/I"="A", "R/W"="R", "chan"=1, "val (float)"=0.0}  # Tx msg cluster
              # "values not expected in 'normal' operating conditions"
              # "Get temperature (deg C)"
              n177 = To Unsigned Byte Integer(number=w524) -> (unsigned 8bit integer=w531:u8)
              n178 = To Unsigned Byte Integer(number=w525) -> (unsigned 8bit integer=w529:u8)
              n179 = Bundle By Name(cluster=w526, "dest"=w531, "A/D/C/I"="T" ("A/D"), "R/W"="R", "chan"=w529, "val (float)"=sgl 0.0) -> (w522:T12)
              n180 = call "Arduino generic wrapper.vi"("Tx msg cluster"=w522, "Channel Name"=w507, "Port name"=w523) -> ("Scan comment"=w512:string, "Output"=w510:dbl)
              n181 = Empty String/Path?(string/path=w512) -> (empty?=w511:bool)
              n182 = Select(t=w510, s=w511, f=w508) -> (s? t:f=w509:dbl)
              n183 = Less?(x=w510, y=-40.0) -> (x < y?=w513:bool)
              n184 = Greater?(x=w510, y=140.0) -> (0:w514:bool)
              n185 = case shown="False" w513 {
                tunnel: [w533 "Faulty thermistor open-circuit;"] -> w515
                tunnel: w514 -> [w532 _]
                frame False {
                  n186 = case shown="True" w532 {
                    tunnel: ["" "Faulty thermistor short-circuit;"] -> w533
                    frame False {
                    }
                    frame True {
                    }
                  }
                }
                frame True {
                }
              }
              n187 = Or(x=w513, y=w514) -> (x .or. y?=w518:bool)
              n188 = Select(t=nan ("f"), s=w518, f=w509) -> (s? t:f=w521:dbl)
              n189 = Concatenate Strings(w512, w515) -> (w516:string)
            }
            frame 2 {
              w547 = T12 {"dest"=1, "A/D/C/I"="A", "R/W"="R", "chan"=1, "val (float)"=0.0}  # Tx msg cluster
              # "Get relative humidity (%)"
              n190 = To Unsigned Byte Integer(number=w545) -> (unsigned 8bit integer=w552:u8)
              n191 = To Unsigned Byte Integer(number=w546) -> (unsigned 8bit integer=w550:u8)
              n192 = Bundle By Name(cluster=w547, "dest"=w552, "A/D/C/I"="H" ("A/D"), "R/W"="R", "chan"=w550, "val (float)"=sgl 0.0) -> (w543:T12)
              n193 = call "Arduino generic wrapper.vi"("Tx msg cluster"=w543, "Channel Name"=w537, "Port name"=w544) -> ("Scan comment"=w540:string, "Output"=w539:dbl)
              n194 = Empty String/Path?(string/path=w540) -> (empty?=w542:bool)
              n195 = Select(t=w539, s=w542, f=w541) -> (s? t:f=w538:dbl)
            }
            frame 3 {
              w563 = T12 {"dest"=1, "A/D/C/I"="A", "R/W"="R", "chan"=1, "val (float)"=0.0}  # Tx msg cluster
              # "Get fluid property"
              n196 = To Unsigned Byte Integer(number=w561) -> (unsigned 8bit integer=w568:u8)
              n197 = To Unsigned Byte Integer(number=w562) -> (unsigned 8bit integer=w566:u8)
              n198 = Bundle By Name(cluster=w563, "dest"=w568, "A/D/C/I"="R" ("A/D"), "R/W"="R", "chan"=w566, "val (float)"=sgl 0.0) -> (w559:T12)
              n199 = call "Arduino generic wrapper.vi"("Tx msg cluster"=w559, "Channel Name"=w553, "Port name"=w560) -> ("Scan comment"=w556:string, "Output"=w555:dbl)
              n200 = Empty String/Path?(string/path=w556) -> (empty?=w558:bool)
              n201 = Select(t=w555, s=w558, f=w557) -> (s? t:f=w554:dbl)
            }
            frame 4 {
              w579 = T12 {"dest"=1, "A/D/C/I"="A", "R/W"="R", "chan"=1, "val (float)"=0.0}  # Tx msg cluster
              # "Get flow speed (m/s). Time-averaged between calls."
              n202 = To Unsigned Byte Integer(number=w577) -> (unsigned 8bit integer=w584:u8)
              n203 = To Unsigned Byte Integer(number=w578) -> (unsigned 8bit integer=w582:u8)
              n204 = Bundle By Name(cluster=w579, "dest"=w584, "A/D/C/I"="U" ("A/D"), "R/W"="R", "chan"=w582, "val (float)"=sgl 0.0) -> (w575:T12)
              n205 = call "Arduino generic wrapper.vi"("Tx msg cluster"=w575, "Channel Name"=w569, "Port name"=w576) -> ("Scan comment"=w572:string, "Output"=w571:dbl)
              n206 = Empty String/Path?(string/path=w572) -> (empty?=w574:bool)
              n207 = Select(t=w571, s=w574, f=w573) -> (s? t:f=w570:dbl)
            }
            frame 5 {
              w595 = T12 {"dest"=1, "A/D/C/I"="A", "R/W"="R", "chan"=1, "val (float)"=0.0}  # Tx msg cluster
              # "Get IMU value"
              n208 = To Unsigned Byte Integer(number=w593) -> (unsigned 8bit integer=w600:u8)
              n209 = To Unsigned Byte Integer(number=w594) -> (unsigned 8bit integer=w598:u8)
              n210 = Bundle By Name(cluster=w595, "dest"=w600, "A/D/C/I"="X" ("A/D"), "R/W"="R", "chan"=w598, "val (float)"=sgl 0.0) -> (w591:T12)
              n211 = call "Arduino generic wrapper.vi"("Tx msg cluster"=w591, "Channel Name"=w585, "Port name"=w592) -> ("Scan comment"=w588:string, "Output"=w587:dbl)
              n212 = Empty String/Path?(string/path=w588) -> (empty?=w590:bool)
              n213 = Select(t=w587, s=w590, f=w589) -> (s? t:f=w586:dbl)
            }
            frame Default {
              # "N.B. all fluid properties (sub 3) are evaluated at T_film"
              # "Oh dear, user has created a server channel with an invalid \"sub\" address"
            }
          }
        }
        frame "ClimatronicsUDP" {
          # "Climatronics sonic anemometer thru Serial to Ether converter"
          n214 = call "ClimatronicsUDP_get_rdg.vi"("Address"=w603) -> ("Output"=w604:dbl, "Status note"=w605:string)  [unwired: 5 in]
        }
        frame "MoconTCP" {
          # "MOCON FID TCP comms"
          n215 = call "MOCON_get_rdg.vi"("Address"=w608) -> ("Output"=w606:dbl, "Status note"=w607:string)  [unwired: 5 in]
        }
        frame "DRUCK" {
        }
        frame "DLI WebPowerSwitch" {
          # "https://www.digital-loggers.com/lpc.html"
          n216 = call "DLIWebPowerSwitch.vi"("Value to Output"=w611, "Ch Description"=w614) -> ("Scan comment"=w612:string, "Output"=w613:dbl)  [unwired: 5 in, 1 out]
        }
        frame "AalborgMFC" {
          n217 = call "AalborgMFC.vi"("Value to Output"=w617, "Ch Description"=w618) -> ("Scan comment"=w616:string, "Output"=w615:dbl)  [unwired: 5 in, 1 out]
        }
        frame "AlicatMFC" {
          n218 = call "AlicatMFC.vi"("Value to Output"=w621, "Ch Description"=w622) -> ("Scan comment"=w620:string, "Reading"=w619:dbl)  [unwired: 5 in, 1 out]
        }
        frame "GILL" {
          n219 = call "Gill_get_rdg.vi"("Channel Name"=w624, "Address"=w623) -> ("Output"=w626:dbl, "Status note"=w625:string)  [unwired: 2 in, 2 out]
        }
        frame "IR2100" {
          n220 = call "IR2100_get_rdg.vi"("Address"=w627) -> ("Comment"=w629:string, "Reading"=w628:dbl)  [unwired: 2 in, 2 out]
        }
        frame "JEM" {
          n221 = Unbundle By Name(w646) -> ("Main"=w632:i32, "Ch."=w631:i32, "Port Name"=w641:string)
          n222 = case shown="0, Default" w631 {
            tunnel: [i16[] [-3, -2, -1, 0, 14, 29, 43, 57, 71, 86, 100] i16[] [0, 20, 40, 60, 80, 100, 120]] -> w635
            tunnel: [u8[] [10, 50, 80, 100, 120, 140, 160, 180, 200, 220, 240] u8[] [20, 50, 90, 130, 160, 200, 230]] -> w636
            frame 0, Default {
            }
            frame 1 {
            }
          }
          n223 = Add(x=w632, y=w631) -> (x+y=w630:i32)
          n224 = Threshold 1D Array(2:w642, 3:w635) -> (0:w638:dbl)  [unwired: 1 out]
          n225 = Round To Nearest(number=w638) -> (nearest integer value=w639:dbl)
          n226 = To Long Integer(number=w639) -> (32bit integer=w637:i32)
          n227 = Index Array(array=w636, index=w637) -> (element=w634:u8)
          n228 = call "DMX.vi"("Port Name"=w641, "DMX channel no."=w630, "Set value:"=w634, "Channel Name"=w645) -> ("error"=w640:bool)  [unwired: 2 out]
          n229 = Index Array(array=w635, index=w637) -> (element=w633:i16)
          n230 = case shown="False" w640 {
            tunnel: [w647 nan] -> w644
            tunnel: ["" "Comms Error"] -> w643
            tunnel: w633 -> [w649 _]
            frame False {
              n231 = To Double Precision Float(number=w649) -> (double precision float=w647:dbl)
            }
            frame True {
            }
          }
        }
        frame "LabJack T7" {
          # "Type : LabJack T7 is used to read & write high level IO. The T7 has AIN#(0:14), AOUT#(0:1), DIO#(0:22)"
          n232 = call "T7-BasicModbusIO.vi"("MaxAge(s)"=w656, "Value to Output"=w660, "Ch Description"=w659) -> ("upper limit"=w658:dbl, "String"=w657:string)  [unwired: 7 in]
        }
        frame "LabJack T7 MODBUS" {
          # "Type : LabJack T7 MODBUS  = access to the MODBUS Map registers. Consult T7 Datasheet for target register description."
          n233 = call "T7-FullModbus.vi"("MaxAge(s)"=w661, "Value to Output"=w664, "Ch Description"=w665) -> ("Output Value"=w662:dbl, "String"=w663:string)  [unwired: 7 in]
        }
        frame "LPA" {
          # "LPA was, IIRC, a serially-polled weighing platform we rented at Surrey for Athena Scaperdas' project at Atkins to weigh a helicopter with rotor running. \nTo add to the fun, it was RS232, so to make it addressable it was polled through an addressable ADAM 485-232 module"
          n234 = call "LPA400_get_rdg.vi"("Channel Name"=w668, "Address"=w669) -> ("Output"=w666:dbl, "Status note"=w667:string)  [unwired: 4 out]
        }
        frame "PPT" {
          n235 = call "PPT_get_rdg.vi"("Channel Name"=w671, "Address"=w670) -> ("Reading"=w673:dbl, "Comment"=w672:string)  [unwired: 2 in, 2 out]
        }
        frame "Thermistor" {
          # "Could be replaced with use of an \"Equation\" channel..."
          n236 = call "4017_18_get_rdg.vi"("Channel Name"=w677, "Address"=w676) -> ("Reading"=w675:dbl, "Comment"=w678:string)  [unwired: 2 in, 2 out]
          n237 = call "Thermistor volts to temperature.vi"("V2 (V)"=w675) -> ("Temperature (degC)"=w674:dbl)
        }
        frame "Tracker" {
          # "Intended as a replacement for Gulton-West Octets. Proved to have insoluble problem with CJC when packed in rack."
          n238 = while {
            tunnel: w684 -> [w708]
            tunnel: w683 -> [w707]
            tunnel: [w701] -> w682
            tunnel: w681 -> [w700]
            tunnel: [w694] -> w680
            tunnel: w679 -> [w693]
            i -> [w690]
            stop <- w687 continue-if-true
            n239 = Unbundle By Name(w707) -> ("Function"=w706:T3)
            n240 = Unbundle By Name(w708) -> ("Port Name"=w705:string, "Ch."=w696:i32, "Main"=w704:i32, "Sub"=w703:i32)
            n241 = case shown="\"Analogue Output\"" w706 {
              tunnel: [enum16{"Set", "Read"}."Set" ("Set") enum16{"Set", "Read"}."Set" ("Set") enum16{"Set", "Read"}."Set" ("Set") enum16{"Set", "Read"}."Set" ("Set") enum16{"Set", "Read"}."Set" ("Set") enum16{"Set", "Read"}."Read" ("Set") enum16{"Set", "Read"}."Read" ("Set")] -> w691
              tunnel: [enum16{"Logic", "Analogue"}."Analogue" ("Analogue") enum16{"Logic", "Analogue"}."Logic" ("Analogue") enum16{"Logic", "Analogue"}."Logic" ("Analogue") enum16{"Logic", "Analogue"}."Logic" ("Analogue") enum16{"Logic", "Analogue"}."Logic" ("Analogue") enum16{"Logic", "Analogue"}."Logic" ("Analogue") enum16{"Logic", "Analogue"}."Analogue" ("Analogue")] -> w702
              frame "Analogue Output" {
              }
              frame "Digital Output" {
              }
              frame "Relay Output" {
              }
              frame "Event rate" {
              }
              frame "Event counter" {
              }
              frame "Digital Input" {
              }
              frame "Analogue Input" {
              }
            }
            n242 = call "TalkTracker.vi"("PORT NAME"=w705, "Set"=w691, "Channel Name"=w700, "Value to set"=w693, "MODULE ADDRESS"=w704, "LOCATION"=w696, "NO. LOCATIONS"=w703, "Analogue"=w702) -> ("Response"=w698:string, "Good Set?"=w685:bool, "Comment out"=w701:string)  [unwired: 1 in, 4 out]
            n243 = Match Pattern(string=w698, regular expression="\r\n") -> (before substring=w697:string)  [unwired: 4 out]
            n244 = case shown="\"Set\"" w691 {
              tunnel: w697 -> [_ w720]
              tunnel: [w712 w719] -> w695
              tunnel: w693 -> [w714 _]
              tunnel: nan ("Reading") -> [w713 w718]
              tunnel: [w711 w716] -> w688
              tunnel: [0 ("y") 1 ("y")] -> w686
              tunnel: w685 -> [w709 _]
              frame "Set" {
                n245 = Not(x=w709) -> (.not. x?=w711:bool)
                n246 = Select(t=w714, s=w709, f=w713) -> (s? t:f=w712:dbl)
              }
              frame "Read" {
                n247 = String Length(string=w720) -> (length=w722:i32)
                n248 = Fract/Exp String To Number(string=w720, default (0 dbl)=w718) -> (offset past number=w723:i32, number=w721:dbl)  [unwired: 2 out]
                n249 = Equal?(x=w722, y=w723) -> (x = y?=w717:bool)
                n250 = Not(x=w717) -> (.not. x?=w716:bool)
                n251 = Select(t=w721, s=w717, f=w718) -> (s? t:f=w719:dbl)
              }
            }
            n252 = case shown="283" w696 {
              tunnel: w695 -> [w724 w727]
              tunnel: [w724 w725] -> w694
              frame 0, Default {
              }
              frame 283 {
                n253 = Equal To 0?(x=w727) -> (x = 0?=w728:bool)
                n254 = Select(t=nan ("Reading"), s=w728, f=w727) -> (s? t:f=w725:dbl)
              }
            }
            n255 = Less?(x=w690, y=w686) -> (x < y?=w689:bool)
            n256 = And(x=w688, y=w689) -> (x .and. y?=w687:bool)
          }
        }
        frame "Vaisala" {
          # "Thermo-hygrometer"
          n257 = Unbundle By Name(w749) -> ("Main"=w745:i32, "Ch."=w746:i32, "Port Name"=w747:string)
          n258 = call "HMP231.vi"("Channel Name"=w748, "Port Name"=w747, "Channel"=w746, "Address"=w745) -> ("Output"=w743:dbl, "Status note"=w744:string)  [unwired: 2 out]
        }
        frame "WEST" {
          # "Proposed new mini-DIN PID controllers?"
        }
        frame "X10" {
          (unwired) 1 items=["-----", "A", "B", "C", "D", "E", "F", "G", "H", "I", "J", "K", "L", "M", "N", "O", "P"] ("House Code")
          # "X10 powerline-signalling controller"
          n259 = Greater Than 0?(x=w756) -> (x > 0?=w755:bool)
          n260 = Unbundle By Name(w761) -> ("Port Name"=w758:string, "Main"=w759:i32, "Ch."=w760:i32)
          n261 = call "X10control.vi"("Port Name"=w758, "Power Request (ON)"=w755, "House Code"=w759, "Unit No."=w760) -> ()  [unwired: 6 out]
          n262 = Select(t=1.0, s=w755, f=0.0) -> (s? t:f=w752:dbl)
        }
        frame "VIRTUAL" {
          n263 = case shown="\"GMU:Source:Meas Den Ratio\"" w768 {
            tunnel: [w782 w796 w813 w822 w854 w880 w902 w917 w928 w942 w965 w994 w1077 w1082 w1108 w1137 w1156 w1161 w1237 w1281] -> w772
            tunnel: [w773 w802 w807 w833 w862 w878 w906 w911 w926 w955 w974 w995 w1071 w1081 w1107 "" "" ("Scan comments") w1162 w1238 w1282] -> w771
            tunnel: w770 -> [w779 w804 w810 w834 w863 w884 w908 w913 w931 w953 w976 w997 w1073 w1086 w1111 _ _ w1164 w1240 w1284]
            tunnel: w769 -> [w780 w803 w811 w835 w864 w885 w907 w912 w932 w954 w975 w998 w1072 w1088 w1113 _ _ w1163 w1239 w1283]
            tunnel: w768 -> [w777 _ _ _ _ _ _ _ _ _ _ _ _ _ _ w1132 _ _ _ _]
            tunnel: w767 -> [w778 _ _ _ _ _ _ _ _ _ _ _ _ w1079 w1106 w1137 _ w1160 w1236 w1280]
            tunnel: w766 -> [w781 _ _ _ _ _ _ _ _ _ _ _ _ w1083 w1109 _ _ w1159 w1235 w1279]
            tunnel: w765 -> [_ _ _ _ _ w876 _ _ _ _ _ w999 _ _ _ _ _ _ _ _]
            tunnel: w764 -> [_ w795 w812 _ _ _ _ _ w925 _ _ _ _ _ _ _ _ _ _ _]
            tunnel: w763 -> [_ _ _ _ _ _ _ _ _ _ _ _ _ _ _ _ _ _ _ _]
            tunnel: w762 -> [_ _ _ _ _ _ _ _ _ _ _ w992 _ _ _ _ _ _ _ _]
            frame "GMU:Remaining:", Default {
              n264 = Match Pattern(string=w777, regular expression="GMU:Remaining:" ("String to match")) -> (match substring=w775:string)  [unwired: 4 out]
              n265 = Empty String/Path?(string/path=w775) -> (empty?=w774:bool)
              n266 = case shown="False" w774 {
                tunnel: [w789 nan] -> w782
                tunnel: w781 -> [w788 _]
                tunnel: w780 -> [w787 _]
                tunnel: w779 -> [w786 _]
                tunnel: w778 -> [w785 _]
                tunnel: w777 -> [w784 _]
                tunnel: [w783 w791] -> w773
                frame False {
                  n267 = call "Update_Rem_gas.vi"("Scan Period (s)"=w785, "Gas Remaining in"=w788, "Ch name"=w784, "Ch names"=w786, "Present scan array"=w787) -> ("Gas Remaining out"=w789:dbl, "Comments"=w783:string)  [unwired: 1 out]
                }
                frame True {
                  n268 = Current VI's Path() -> (path=w793:path)
                  n269 = Path To String(path=w793) -> (string=w792:string)
                  n270 = Concatenate Strings(" was not matched in ", w792) -> (w791:string)
                }
              }
            }
            frame "GMU:Source:Meas Q" {
              n271 = call "Calculate_Release_Flowrates.vi"("Ch names"=w804, "Units"=enum16{"Q l/min", "M_dot Kg/min"}."Q l/min", "Present scan array"=w803) -> ("Trace"=w800:dbl, "Carrier"=w801:dbl, "Scan comments"=w802:string)
              n272 = Add(x=w801, y=w800) -> (x+y=w797:dbl)
              n273 = Not Equal To 0?(x=w797) -> (x != 0?=w798:bool)
              n274 = Select(t=w797, s=w798, f=w795) -> (s? t:f=w796:dbl)
            }
            frame "GMU2:Source:Meas Q" {
              n275 = call "GMU2 Channel Names.vi"() -> ("GMU2 Source Channels"=w806:string[])  [unwired: 10 in, 1 out]
              n276 = for {
                tunnel: w806 -> [w817] mode=indexing
                tunnel: [w816] -> w805 mode=indexing
                n277 = Concatenate Strings(w817, "Meas Q" ("string")) -> (w816:string)
              }
              n278 = call "Read_Earlier_Channels.vi"("Present scan array"=w811, "Ch names"=w810, "Desired Channels"=w805) -> ("Scan comments"=w807:string, "Index 0"=w809:dbl, "Index 1"=w808:dbl)  [unwired: 3 out]
              n279 = Add(x=w809, y=w808) -> (x+y=w814:dbl)
              n280 = Not Equal To 0?(x=w814) -> (x != 0?=w815:bool)
              n281 = Select(t=w814, s=w815, f=w812) -> (s? t:f=w813:dbl)
            }
            frame "GMU2:Source:Meas Strength" {
              n282 = call "GMU2 Channel Names.vi"() -> ("GMU2 Source Channels"=w820:string[])  [unwired: 10 in, 1 out]
              n283 = for {
                tunnel: w820 -> [w837] mode=indexing
                tunnel: [w836] -> w819 mode=indexing
                n284 = Concatenate Strings(w837, "Meas Q" ("string")) -> (w836:string)
              }
              n285 = call "Read_Earlier_Channels.vi"("Present scan array"=w835, "Ch names"=w834, "Desired Channels"=w819) -> ("Scan comments"=w833:string, "Index 0"=w824:dbl, "Index 1"=w823:dbl)  [unwired: 3 out]
              n286 = Equal To 0?(x=w824) -> (x = 0?=w831:bool)
              n287 = Equal To 0?(x=w823) -> (x = 0?=w832:bool)
              n288 = And(x=w831, y=w832) -> (x .and. y?=w830:bool)
              n289 = case shown="False" w830 {
                tunnel: w824 -> [w849 _]
                tunnel: w823 -> [w848 _]
                tunnel: [w847 0.0] -> w821
                frame False {
                  n290 = Add(x=w849, y=w848) -> (x+y=w852:dbl)
                  n291 = Divide(x=w848, y=w852) -> (x/y=w851:dbl)
                  n292 = Multiply(x=w851, y=100.0) -> (x*y=w847:dbl)
                }
                frame True {
                }
              }
              n293 = while {
                tunnel: [w840] -> w825
                tunnel: [w841] -> w827
                tunnel: w821 -> [w846]
                shift-left: _ -> [w840]
                shift-left: _ -> [w845]
                shift-right: [w846] -> _
                stop <- FALSE continue-if-true
                w844 = 6.0 ("y")
                n294 = Less?(x=w845, y=w844) -> (x < y?=w843:bool)
                n295 = Less?(x=w840, y=w844) -> (x < y?=w842:bool)
                n296 = Or(x=w843, y=w842) -> (x .or. y?=w841:bool)
              }
              n297 = Greater?(x=w821, y=7.0) -> (0:w826:bool)
              n298 = And(x=w827, y=w826) -> (x .and. y?=w828:bool)
              n299 = Select(t=w825, s=w828, f=w821) -> (s? t:f=w822:dbl)
            }
            frame "GMU2:Calib:Meas ppm" {
              n300 = call "GMU2 Channel Names.vi"() -> ("GMU2 Calib Channels"=w855:string[])  [unwired: 10 in, 1 out]
              n301 = for {
                tunnel: w855 -> [w866] mode=indexing
                tunnel: [w865] -> w856 mode=indexing
                n302 = Concatenate Strings(w866, "Meas Q" ("string")) -> (w865:string)
              }
              n303 = call "Read_Earlier_Channels.vi"("Present scan array"=w864, "Ch names"=w863, "Desired Channels"=w856) -> ("Scan comments"=w862:string, "Index 0"=w858:dbl, "Index 1"=w857:dbl)  [unwired: 3 out]
              n304 = Equal To 0?(x=w858) -> (x = 0?=w860:bool)
              n305 = Equal To 0?(x=w857) -> (x = 0?=w861:bool)
              n306 = And(x=w860, y=w861) -> (x .and. y?=w859:bool)
              n307 = case shown="False" w859 {
                tunnel: w858 -> [w870 _]
                tunnel: w857 -> [w869 _]
                tunnel: [w868 0.0] -> w854
                frame False {
                  n308 = Add(x=w870, y=w869) -> (x+y=w873:dbl)
                  n309 = Divide(x=w869, y=w873) -> (x/y=w872:dbl)
                  n310 = Multiply(x=w872, y=1000000.0) -> (x*y=w868:dbl)
                }
                frame True {
                }
              }
            }
            frame "GMU:Detector:Strength" {
              n311 = Unbundle By Name(w876) -> ("C"=w875:dbl)
              n312 = call "Read_value_of_earlier_Ch.vi"("Desired Ch to Read"="GMU:Detector:Meas Current", "Ch names"=w884, "Present scan array"=w885) -> ("Value"=w881:dbl, "Scan comment"=w879:string)  [unwired: 1 in]
              n313 = Greater?(x=w881, y=w875) -> (0:w882:bool)
              n314 = case shown="True" w882 {
                tunnel: w876 -> [_ w897]
                tunnel: w881 -> [_ w892]
                tunnel: [100.0 ("Eng Values") w890] -> w880
                tunnel: ["Fault" w893] -> w877
                frame False {
                }
                frame True {
                  n315 = Unbundle By Name(w897) -> ("D"=w888:dbl, "A"=w896:dbl, "B"=w895:dbl)
                  n316 = Less?(x=w892, y=w888) -> (x < y?=w891:bool)
                  n317 = Build Array(w896, w895) -> (w894:dbl[])
                  n318 = call "Polynomial_convert.vi"("Calib constants"=w894, "Voltage"=w892) -> ("Eng Values"=w889:dbl)  [unwired: 4 out]
                  n319 = case shown="True" w891 {
                    tunnel: ["Saturated" ""] -> w893
                    tunnel: [100.0 ("Eng Values") w900] -> w890
                    tunnel: w889 -> [_ w900]
                    frame False {
                    }
                    frame True {
                    }
                  }
                }
              }
              n320 = Concatenate Strings(w879, w877) -> (w878:string)
            }
            frame "GMU:Source:Meas M_dot" {
              n321 = call "Calculate_Release_Flowrates.vi"("Ch names"=w908, "Units"=enum16{"Q l/min", "M_dot Kg/min"}."M_dot Kg/min", "Present scan array"=w907) -> ("Trace"=w904:dbl, "Carrier"=w905:dbl, "Scan comments"=w906:string)
              n322 = Add(x=w905, y=w904) -> (x+y=w902:dbl)
            }
            frame "GMU:Source:Meas Density" {
              n323 = Build Array("GMU:Source:Meas M_dot", "GMU:Source:Meas Q") -> (w914:string[])
              n324 = call "Read_Earlier_Channels.vi"("Present scan array"=w912, "Ch names"=w913, "Desired Channels"=w914) -> ("Scan comments"=w911:string, "Index 0"=w910:dbl, "Index 1"=w909:dbl)  [unwired: 3 out]
              n325 = Not Equal To 0?(x=w910) -> (x != 0?=w918:bool)
              n326 = case shown="False" w918 {
                tunnel: w910 -> [_ w922]
                tunnel: w909 -> [_ w921]
                tunnel: [0.0 w920] -> w917
                frame False {
                }
                frame True {
                  n327 = Divide(x=w922, y=w921) -> (x/y=w923:dbl)
                  n328 = Multiply(x=w923, y=1000.0) -> (x*y=w920:dbl)
                }
              }
            }
            frame "GMU:Source:Meas Den Ratio" {
              n329 = call "Read_value_of_earlier_Ch.vi"("Desired Ch to Read"="GMU:Source:Meas Density", "Ch names"=w931, "Present scan array"=w932) -> ("Value"=w927:dbl, "Scan comment"=w926:string)  [unwired: 1 in]
              n330 = Equal?(x=w927, y=w925) -> (x = y?=w929:bool)
              n331 = case shown="False" w929 {
                tunnel: w927 -> [w934 _]
                tunnel: [w933 w939] -> w928
                tunnel: w925 -> [_ w939]
                frame False {
                  n332 = global read "Gas_management_global.vi" "GMU1 Release temp (deg C)"() -> (w937:dbl)
                  n333 = global read "Gas_management_global.vi" "Atmos Pres (mbars)"() -> (w936:dbl)
                  n334 = call "Gas_Density.vi"("Pressure (mbar)"=w936, "Temperature (C)"=w937, "Gas"="Air" ("Gas Name")) -> ("Density (kg/m^3) (= g/l)"=w935:dbl)
                  n335 = Divide(x=w934, y=w935) -> (x/y=w933:dbl)
                }
                frame True {
                }
              }
            }
            frame "GMU:Source:ppm/%Density" {
              # "Source ppm"
              # "% Delta Density of source"
              n336 = call "Read_value_of_earlier_Ch.vi"("Desired Ch to Read"="GMU:Source:Meas Strength", "Ch names"=w953, "Present scan array"=w954) -> ("Value"=w951:dbl, "Scan comment"=w955:string)  [unwired: 1 in]
              n337 = call "Read_value_of_earlier_Ch.vi"("Desired Ch to Read"="GMU:Source:Meas Den Ratio", "Ch names"=w953, "Present scan array"=w954) -> ("Value"=w949:dbl)  [unwired: 1 in, 1 out]
              n338 = Subtract(x=w949, y=1.0) -> (x-y=w946:dbl)
              n339 = Multiply(x=w951, y=10000.0) -> (x*y=w947:dbl)
              n340 = Multiply(x=w946, y=100.0) -> (x*y=w940:dbl)
              n341 = Absolute Value(x=w940) -> (abs(x)=w941:dbl)
              n342 = Greater?(x=w941, y=1.5) -> (0:w943:bool)
              n343 = case shown="False" w943 {
                tunnel: w947 -> [_ w960]
                tunnel: w940 -> [_ w959]
                tunnel: [nan w958] -> w942
                frame False {
                }
                frame True {
                  n344 = Divide(x=w960, y=w959) -> (x/y=w958:dbl)
                }
              }
            }
            frame "GMU:Source:Meas Strength" {
              n345 = call "Calculate_Release_Flowrates.vi"("Ch names"=w976, "Units"=enum16{"Q l/min", "M_dot Kg/min"}."Q l/min", "Present scan array"=w975) -> ("Trace"=w968:dbl, "Carrier"=w969:dbl, "Scan comments"=w974:string)
              n346 = Equal To 0?(x=w969) -> (x = 0?=w971:bool)
              n347 = Equal To 0?(x=w968) -> (x = 0?=w972:bool)
              n348 = And(x=w971, y=w972) -> (x .and. y?=w970:bool)
              n349 = case shown="False" w970 {
                tunnel: w969 -> [w987 _]
                tunnel: w968 -> [w986 _]
                tunnel: [w985 0.0] -> w964
                frame False {
                  n350 = Add(x=w987, y=w986) -> (x+y=w990:dbl)
                  n351 = Divide(x=w986, y=w990) -> (x/y=w989:dbl)
                  n352 = Multiply(x=w989, y=100.0) -> (x*y=w985:dbl)
                }
                frame True {
                }
              }
              n353 = while {
                tunnel: [w978] -> w961
                tunnel: [w979] -> w963
                tunnel: w964 -> [w984]
                shift-left: _ -> [w978]
                shift-left: _ -> [w983]
                shift-right: [w984] -> _
                stop <- FALSE continue-if-true
                w982 = 6.0 ("y")
                n354 = Less?(x=w983, y=w982) -> (x < y?=w981:bool)
                n355 = Less?(x=w978, y=w982) -> (x < y?=w980:bool)
                n356 = Or(x=w981, y=w980) -> (x .or. y?=w979:bool)
              }
              n357 = Greater?(x=w964, y=7.0) -> (0:w962:bool)
              n358 = And(x=w963, y=w962) -> (x .and. y?=w966:bool)
              n359 = Select(t=w961, s=w966, f=w964) -> (s? t:f=w965:dbl)
            }
            frame "EnFlo_Tunnel:Inlet_Temp:St Deviation" {
              n360 = global read "ADAM_Global.vi" "Active Ch names"() -> (w1003:string[])
              n361 = Unbundle By Name(w999) -> ("A"=w1000:dbl)
              n362 = Less?(x=w1000, y=2.0) -> (x < y?=w1001:bool)
              n363 = case shown="False" w1001 {
                tunnel: w997 -> [_ w1038]
                tunnel: w998 -> [_ w1037]
                tunnel: string[] ["EnFlo_Tunnel:Inlet_Y=-1500:Z=50", "EnFlo_Tunnel:Inlet_Y=-1000:Z=50", "EnFlo_Tunnel:Inlet_Y=-500:Z=50", "EnFlo_Tunnel:Temp:Inlet_15_Bottom", "EnFlo_Tunnel:Inlet_Y=500:Z=50", "EnFlo_Tunnel:Inlet_Y=1000:Z=50", "EnFlo_Tunnel:Inlet_Y=1500:Z=50", "EnFlo_Tunnel:Inlet_Y=-1500:Z=450", "EnFlo_Tunnel:Inlet_Y=-1000:Z=450", "EnFlo_Tunnel:Inlet_Y=-500:Z=450", "EnFlo_Tunnel:Temp:Inlet_11", "EnFlo_Tunnel:Inlet_Y=500:Z=450", "EnFlo_Tunnel:Inlet_Y=1000:Z=450", "EnFlo_Tunnel:Inlet_Y=1500:Z=450", "EnFlo_Tunnel:Inlet_Y=-1500:Z=950", "EnFlo_Tunnel:Inlet_Y=-1000:Z=950", "EnFlo_Tunnel:Inlet_Y=-500:Z=950", "EnFlo_Tunnel:Temp:Inlet_6", "EnFlo_Tunnel:Inlet_Y=500:Z=950", "EnFlo_Tunnel:Inlet_Y=1000:Z=950", "EnFlo_Tunnel:Inlet_Y=1500:Z=950", "EnFlo_Tunnel:Inlet_Y=-1500:Z=1450", "EnFlo_Tunnel:Inlet_Y=-1000:Z=1450", "EnFlo_Tunnel:Inlet_Y=-500:Z=1450", "EnFlo_Tunnel:Temp:Inlet_1_Top", "EnFlo_Tunnel:Inlet_Y=500:Z=1450", "EnFlo_Tunnel:Inlet_Y=1000:Z=1450", "EnFlo_Tunnel:Inlet_Y=1500:Z=1450", "EnFlo_Tunnel:Setpoint:Inlet_15_Bottom", "EnFlo_Tunnel:Setpoint:Inlet_11", "EnFlo_Tunnel:Setpoint:Inlet_6", "EnFlo_Tunnel:Setpoint:Inlet_1_Top"] ("subarray") -> [w1009 w1036]
                tunnel: [w1007 w1034] -> w995
                tunnel: w1003 -> [_ w1033]
                tunnel: [w1010 w1030] -> w993
                tunnel: w1000 -> [w1011 _]
                tunnel: w992 -> [w1004 _]
                frame False {
                  w1017 = FALSE  # All Active Channels
                  n364 = Subtract(x=w1004, y=w1011) -> (x-y=w1018:dbl)
                  n365 = call "Get_ADAM_averages_server.vi"("No of averages"=1, "All Active Channels"=w1017, "End time"=w1004, "Start time"=w1018, "Clients time"=w1004, "ADAM Ch Names"=w1009) -> ("DBL values"=w1015:dbl[][])  [unwired: 4 out]
                  n366 = Index Array(array=w1015, index (row)=0) -> (element=w1012:dbl[])  [unwired: 1 in]
                  n367 = Array Subset(array=w1012, index=1) -> (w1006:dbl[])  [unwired: 1 in]
                  n368 = call "Normalise Inlet Temps array.vi"("Temps plus setpoints"=w1006) -> ("Normalised Temps"=w1005:dbl[])
                  n369 = for {
                    tunnel: w1005 -> [w1024] mode=indexing
                    tunnel: [w1024] -> w1010 mode=indexing if=w1022
                    tunnel: w1009 -> [w1021] mode=indexing
                    shift-right: [w1019] -> w1007
                    shift-left: "" -> [w1020]
                    n370 = Not A Number/Path/Refnum?(number/path/refnum=w1024) -> (NaN/Path/Refnum?=w1023:bool)
                    n371 = Not(x=w1023) -> (.not. x?=w1022:bool)
                    n372 = case shown="False" w1022 {
                      tunnel: w1021 -> [w1027 _]
                      tunnel: w1020 -> [w1026 w1029]
                      tunnel: [w1025 w1029] -> w1019
                      frame False {
                        n373 = Format Into String(format string="Channel \"%s\" is not currently active.\n", initial string=w1026, w1027) -> (resulting string=w1025:string)  [unwired: 1 in, 1 out]
                      }
                      frame True {
                      }
                    }
                  }
                }
                frame True {
                  n374 = for {
                    tunnel: w1038 -> [w1052]
                    tunnel: w1037 -> [w1051]
                    tunnel: w1036 -> [w1048] mode=indexing
                    shift-right: [w1049] -> w1034
                    shift-left: "" -> [w1050]
                    tunnel: w1033 -> [w1043]
                    tunnel: [w1042] -> w1032 mode=indexing
                    n375 = call "Read_value_of_earlier_Ch.vi"("Desired Ch to Read"=w1048, "Ch names"=w1052, "Present scan array"=w1051) -> ("Value"=w1046:dbl, "Scan comment"=w1045:string)  [unwired: 1 in]
                    n376 = Not A Number/Path/Refnum?(number/path/refnum=w1046) -> (NaN/Path/Refnum?=w1047:bool)
                    n377 = case shown="False" w1047 {
                      tunnel: w1048 -> [w1055 _]
                      tunnel: [w1058 w1068] -> w1042
                      tunnel: w1046 -> [w1057 w1068]
                      tunnel: [w1060 w1067] -> w1044
                      tunnel: w1045 -> [w1059 w1067]
                      tunnel: w1043 -> [w1056 _]
                      frame False {
                        n378 = Search 1D Array(1D array=w1056, element=w1055) -> (index of element=w1053:i32)  [unwired: 1 in]
                        n379 = Greater Or Equal To 0?(x=w1053) -> (x >= 0?=w1054:bool)
                        n380 = case shown="False" w1054 {
                          tunnel: w1055 -> [w1064 _]
                          tunnel: [w1063 w1066] -> w1060
                          tunnel: w1059 -> [_ w1066]
                          tunnel: [nan w1065] -> w1058
                          tunnel: w1057 -> [_ w1065]
                          frame False {
                            n381 = Format Into String(format string="Channel \"%s\" is not currently active.\n", w1064) -> (resulting string=w1063:string)  [unwired: 2 in, 1 out]
                          }
                          frame True {
                          }
                        }
                      }
                      frame True {
                      }
                    }
                    n382 = Concatenate Strings(w1050, w1044) -> (w1049:string)
                  }
                  n383 = call "Normalise Inlet Temps array.vi"("Temps plus setpoints"=w1032) -> ("Normalised Temps"=w1031:dbl[])
                  n384 = for {
                    tunnel: w1031 -> [w1040] mode=indexing
                    tunnel: [w1040] -> w1030 mode=indexing if=w1039
                    n385 = Not A Number/Path/Refnum?(number/path/refnum=w1040) -> (NaN/Path/Refnum?=w1041:bool)
                    n386 = Not(x=w1041) -> (.not. x?=w1039:bool)
                  }
                }
              }
              n387 = call <vilib>:"Std Deviation and Variance.vi"("X"=w993) -> ("standard deviation"=w994:dbl)  [unwired: 1 in, 2 out]
            }
            frame "EnFlo Lab:labstrat1:Delta T" {
              n388 = Build Array("EnFlo Lab:labstrat1:Z=4.5m", "EnFlo Lab:labstrat1:Z=0.5m") -> (w1076:string[])
              n389 = call "Read_Earlier_Channels.vi"("Present scan array"=w1072, "Ch names"=w1073, "Desired Channels"=w1076) -> ("Scan comments"=w1071:string, "Index 0"=w1070:dbl, "Index 1"=w1069:dbl)  [unwired: 3 out]
              n390 = Subtract(x=w1070, y=w1069) -> (x-y=w1077:dbl)
            }
            frame "EnFlo_Tunnel:Hydrosonic:Integral" {
              n391 = Build Array("EnFlo_Tunnel:Reference:Velocity", "Hydrosonic:Transducer:Setting") -> (w1087:string[])
              n392 = call "Read_Earlier_Channels.vi"("Present scan array"=w1088, "Ch names"=w1086, "Desired Channels"=w1087) -> ("Scan comments"=w1081:string, "Index 0"=w1085:dbl, "Index 1"=w1080:dbl)  [unwired: 3 out]
              n393 = global read "EnFlo_Tunnel_Global.vi" "Minimum Ref Velocity"() -> (w1078:dbl)
              n394 = Greater?(x=w1085, y=w1078) -> (0:w1084:bool)
              n395 = case shown="True" w1084 {
                tunnel: w1083 -> [w1091 w1099]
                tunnel: [w1091 w1098] -> w1082
                tunnel: w1080 -> [_ w1097]
                tunnel: w1079 -> [_ w1096]
                frame False {
                }
                frame True {
                  w1094 = 8640000.0  # Seconds per day x 100
                  n396 = Multiply(x=w1097, y=w1096) -> (x*y=w1095:dbl)
                  n397 = Divide(x=w1095, y=w1094) -> (x/y=w1093:dbl)
                  n398 = Not A Number/Path/Refnum?(number/path/refnum=w1093) -> (NaN/Path/Refnum?=w1092:bool)
                  n399 = case shown="False" w1092 {
                    tunnel: w1099 -> [w1102 w1103]
                    tunnel: [w1101 w1103] -> w1098
                    tunnel: w1093 -> [w1100 _]
                    frame False {
                      n400 = Add(x=w1100, y=w1102) -> (x+y=w1101:dbl)
                    }
                    frame True {
                    }
                  }
                }
              }
            }
            frame "EnFlo_Tunnel:Days Run at:2.5m/s" {
              n401 = Build Array("EnFlo_Tunnel:Reference:Velocity") -> (w1112:string[])
              n402 = call "Read_Earlier_Channels.vi"("Present scan array"=w1113, "Ch names"=w1111, "Desired Channels"=w1112) -> ("Scan comments"=w1107:string, "Index 0"=w1105:dbl)  [unwired: 4 out]
              n403 = global read "EnFlo_Tunnel_Global.vi" "Minimum Ref Velocity"() -> (w1104:dbl)
              n404 = Greater?(x=w1105, y=w1104) -> (0:w1110:bool)
              n405 = case shown="True" w1110 {
                tunnel: w1109 -> [w1115 w1123]
                tunnel: [w1115 w1122] -> w1108
                tunnel: w1105 -> [_ w1121]
                tunnel: w1106 -> [_ w1120]
                frame False {
                }
                frame True {
                  w1118 = 216000.0  # Seconds per day x 2.5
                  n406 = Multiply(x=w1121, y=w1120) -> (x*y=w1119:dbl)
                  n407 = Divide(x=w1119, y=w1118) -> (x/y=w1117:dbl)
                  n408 = Not A Number/Path/Refnum?(number/path/refnum=w1117) -> (NaN/Path/Refnum?=w1116:bool)
                  n409 = case shown="True" w1116 {
                    tunnel: w1123 -> [w1126 w1127]
                    tunnel: [w1125 w1127] -> w1122
                    tunnel: w1117 -> [w1124 _]
                    frame False {
                      n410 = Add(x=w1124, y=w1126) -> (x+y=w1125:dbl)
                    }
                    frame True {
                    }
                  }
                }
              }
            }
            frame "Complete:Scan:Period" {
              n411 = while {
                tunnel: [w1140] -> w1133
                tunnel: [w1147] -> w1135
                shift-left: _ -> [w1147]
                shift-right: [w1148] -> w1136
                tunnel: w1132 -> [w1144]
                tunnel: [w1139] -> w1131
                stop <- FALSE continue-if-true
                w1139 = 10.0 ("Averaging time (mins)")
                n412 = Build Array(w1144) -> (w1143:string[])
                n413 = call "Get_Channel_averages.vi"("Desired Ch Names"=w1143, "Averaging time (mins)"=w1139) -> ("number"=w1142:dbl[])  [unwired: 1 in, 2 out]
                n414 = Index Array(array=w1142, index=0) -> (element=w1140:dbl)
                n415 = Greater?(x=w1140, y=20.0) -> (0:w1148:bool)
              }
              n416 = global read "ADAM_Global.vi" "Scan Index"() -> (w1130:i32)
              n417 = Greater?(x=w1130, y=20) -> (0:w1128:bool)
              n418 = Compound Arithmetic op=AND(w1136, invert w1135, w1128) -> (w1134:bool)
              n419 = case shown="True" w1134 {
                tunnel: w1133 -> [_ w1154]
                tunnel: w1131 -> [_ w1149]
                frame False {
                }
                frame True {
                  n420 = Format Into String(format string="Warning! The average scan period on the ADAM Scan table is %.1f seconds over the last %.0f minutes." ("Format String"), w1154, w1149) -> (resulting string=w1152:string)  [unwired: 2 in, 1 out]
                  n421 = call "Server_Emails.vi"("Message"=w1152, "Contact All clients?"=TRUE, "Subject"="Scan Period") -> ()  [unwired: 2 in, 3 out]
                }
              }
            }
            frame "Scan:Padding:(s)" {
              n422 = global read "ADAM_Global.vi" "Scan:Padding:(ms)"() -> (w1157:i32)
              n423 = Divide(x=w1157, y=1000 ("x")) -> (x/y=w1156:dbl)
            }
            frame "GMU:Source:Est Time" {
              # "NaN's"
              # "Est?"
              # "Inband?"
              n424 = stacked-sequence {
                seq-local: [w1165 _ _ _] -> [_ _ w1209 _]
                seq-local: [_ w1177 _ _] -> [_ _ w1206 _]
                seq-local: [_ w1178 _ _] -> [_ _ w1204 _]
                seq-local: [_ _ w1211 _] -> [_ _ _ w1227]
                seq-local: [w1169 _ _ _] -> [_ _ w1208 _]
                seq-local: [_ w1176 _ _] -> [_ _ _ w1223]
                tunnel: w1164 -> [w1171 w1179 w1214 _]
                tunnel: w1163 -> [w1170 w1180 w1215 _]
                tunnel: [_ _ w1207 _] -> w1162
                tunnel: [_ _ _ w1226] -> w1161
                tunnel: w1160 -> [_ _ _ w1225]
                tunnel: w1159 -> [_ _ _ w1224]
                frame #0 {
                  n425 = Build Array("GMU:Carrier 1:Dem Q", "GMU:Carrier 2:Dem Q", "GMU:Trace:Dem Q") -> (w1172:string[])
                  n426 = call "Read_Earlier_Channels.vi"("Present scan array"=w1170, "Ch names"=w1171, "Desired Channels"=w1172) -> ("Scan comments"=w1169:string, "Index 0"=w1168:dbl, "Index 1"=w1167:dbl, "Index 2"=w1166:dbl)  [unwired: 2 out]
                  n427 = Build Array(w1168, w1167, w1166) -> (w1165:dbl[])
                }
                frame #1 {
                  n428 = for {
                    N: 2 -> [_]
                    tunnel: w1180 -> [w1187]
                    tunnel: w1179 -> [w1188]
                    tunnel: [w1186] -> w1177 mode=indexing
                    tunnel: [w1193] -> w1178 mode=indexing
                    tunnel: [w1192] -> w1176 mode=indexing
                    i -> [w1198]
                    w1197 = 10.0  # %
                    n429 = case shown="0, Default" w1198 {
                      tunnel: ["GMU:Source:Meas Q" "GMU:Source:Meas Strength"] -> w1191
                      tunnel: ["GMU:Source:Dem Q" "GMU:Source:Dem Strength"] -> w1190
                      frame 0, Default {
                      }
                      frame 1 {
                      }
                    }
                    n430 = Build Array(w1190, w1191) -> (w1189:string[])
                    n431 = call "Read_Earlier_Channels.vi"("Present scan array"=w1187, "Ch names"=w1188, "Desired Channels"=w1189) -> ("Scan comments"=w1186:string, "Index 0"=w1184:dbl, "Index 1"=w1185:dbl)  [unwired: 3 out]
                    n432 = Not A Number/Path/Refnum?(number/path/refnum=w1185) -> (NaN/Path/Refnum?=w1192:bool)
                    n433 = Greater Than 0?(x=w1184) -> (x > 0?=w1194:bool)
                    n434 = call "In_Range_check.vi"("±"=0.005, "%"=w1197, "Mode"=In_Range."% & ±", "Value"=w1185, "Setpoint"=w1184) -> ("In Range"=w1182:bool)  [unwired: 2 out]
                    n435 = And(x=w1182, y=w1194) -> (x .and. y?=w1195:bool)
                    n436 = Compound Arithmetic op=OR(w1195, invert w1194, w1192) -> (w1193:bool)
                  }
                }
                frame #2 {
                  n437 = while {
                    tunnel: [w1222] -> w1210
                    tunnel: w1209 -> [w1221]
                    shift-left: _ -> [w1222]
                    shift-right: [w1221] -> _
                    stop <- FALSE continue-if-true
                  }
                  n438 = Equal?(x=w1209, y=w1210) -> (x = y?=w1216:bool)
                  n439 = call "Read_value_of_earlier_Ch.vi"("Desired Ch to Read"="GMU:Source:Dem Q", "Ch names"=w1214, "Present scan array"=w1215) -> ("Value"=w1212:dbl)  [unwired: 1 in, 1 out]
                  n440 = Greater Than 0?(x=w1212) -> (x > 0?=w1219:bool)
                  n441 = And Array Elements(Boolean array=w1204) -> (logical AND=w1203:bool)
                  n442 = Select(t=w1203, s=w1219, f=TRUE) -> (s? t:f=w1217:bool)
                  n443 = Compound Arithmetic op=AND(w1216, w1217) -> (w1211:bool)
                  n444 = Concatenate Strings(w1206) -> (w1205:string)
                  n445 = Concatenate Strings(w1205, w1208) -> (w1207:string)
                }
                frame #3 {
                  n446 = case shown="False" w1227 {
                    tunnel: [0.0 w1229] -> w1226
                    tunnel: w1225 -> [_ w1234]
                    tunnel: w1224 -> [_ w1230]
                    tunnel: w1223 -> [_ w1233]
                    frame False {
                    }
                    frame True {
                      n447 = Or Array Elements(Boolean array=w1233) -> (logical OR=w1232:bool)
                      n448 = Add(x=w1234, y=w1230) -> (x+y=w1231:dbl)
                      n449 = Select(t=w1230, s=w1232, f=w1231) -> (s? t:f=w1229:dbl)
                    }
                  }
                }
              }
            }
            frame "GMU2:Source:Est Time" {
              # "NaN's"
              # "Est?"
              n450 = stacked-sequence {
                seq-local: [w1250 _] -> [_ w1271]
                seq-local: [w1244 _] -> [_ w1267]
                tunnel: w1240 -> [w1260 _]
                tunnel: w1239 -> [w1259 _]
                tunnel: [w1243 _] -> w1238
                tunnel: [_ w1270] -> w1237
                tunnel: w1236 -> [_ w1269]
                tunnel: w1235 -> [_ w1268]
                frame #0 {
                  w1254 = 10.0  # %
                  w1257 = 10.0  # %
                  n451 = call "GMU2 Channel Names.vi"() -> ("GMU2 Source Channels"=w1242:string[])  [unwired: 10 in, 1 out]
                  n452 = for {
                    tunnel: w1242 -> [w1264] mode=indexing
                    tunnel: [w1261] -> w1241 mode=concatenating
                    n453 = Concatenate Strings(w1264, "Meas Volts" ("string")) -> (w1263:string)
                    n454 = Concatenate Strings(w1264, "Dem Volts" ("string")) -> (w1262:string)
                    n455 = Build Array(w1262, w1263) -> (w1261:string[])
                  }
                  n456 = call "Read_Earlier_Channels.vi"("Present scan array"=w1259, "Ch names"=w1260, "Desired Channels"=w1241) -> ("Scan comments"=w1243:string, "Index 0"=w1249:dbl, "Index 1"=w1248:dbl, "Index 2"=w1247:dbl, "Index 3"=w1246:dbl)  [unwired: 1 out]
                  n457 = Build Array(w1249, w1248, w1247, w1246) -> (w1245:dbl[])
                  n458 = Not A Number/Path/Refnum?(number/path/refnum=w1245) -> (NaN/Path/Refnum?=w1244:bool[])
                  n459 = call "In_Range_check.vi"("±"=0.005, "%"=w1257, "Mode"=In_Range."% & ±", "Value"=w1248, "Setpoint"=w1249) -> ("In Range"=w1251:bool)  [unwired: 2 out]
                  n460 = call "In_Range_check.vi"("±"=0.005, "%"=w1254, "Mode"=In_Range."% & ±", "Value"=w1246, "Setpoint"=w1247) -> ("In Range"=w1252:bool)  [unwired: 2 out]
                  n461 = And(x=w1251, y=w1252) -> (x .and. y?=w1250:bool)
                }
                frame #1 {
                  n462 = case shown="True" w1271 {
                    tunnel: [0.0 w1273] -> w1270
                    tunnel: w1269 -> [_ w1278]
                    tunnel: w1268 -> [_ w1274]
                    tunnel: w1267 -> [_ w1277]
                    frame False {
                    }
                    frame True {
                      n463 = Or Array Elements(Boolean array=w1277) -> (logical OR=w1276:bool)
                      n464 = Add(x=w1278, y=w1274) -> (x+y=w1275:dbl)
                      n465 = Select(t=w1274, s=w1276, f=w1275) -> (s? t:f=w1273:dbl)
                    }
                  }
                }
              }
            }
            frame "GMU2:Calib:Est Time" {
              # "NaN's"
              # "Est?"
              n466 = stacked-sequence {
                seq-local: [w1294 _] -> [_ w1315]
                seq-local: [w1288 _] -> [_ w1311]
                tunnel: w1284 -> [w1304 _]
                tunnel: w1283 -> [w1303 _]
                tunnel: [w1287 _] -> w1282
                tunnel: [_ w1314] -> w1281
                tunnel: w1280 -> [_ w1313]
                tunnel: w1279 -> [_ w1312]
                frame #0 {
                  w1298 = 10.0  # %
                  w1301 = 10.0  # %
                  n467 = call "GMU2 Channel Names.vi"() -> ("GMU2 Calib Channels"=w1286:string[])  [unwired: 10 in, 1 out]
                  n468 = for {
                    tunnel: w1286 -> [w1308] mode=indexing
                    tunnel: [w1305] -> w1285 mode=concatenating
                    n469 = Concatenate Strings(w1308, "Meas Volts" ("string")) -> (w1307:string)
                    n470 = Concatenate Strings(w1308, "Dem Volts" ("string")) -> (w1306:string)
                    n471 = Build Array(w1306, w1307) -> (w1305:string[])
                  }
                  n472 = call "Read_Earlier_Channels.vi"("Present scan array"=w1303, "Ch names"=w1304, "Desired Channels"=w1285) -> ("Scan comments"=w1287:string, "Index 0"=w1293:dbl, "Index 1"=w1292:dbl, "Index 2"=w1291:dbl, "Index 3"=w1290:dbl)  [unwired: 1 out]
                  n473 = Build Array(w1293, w1292, w1291, w1290) -> (w1289:dbl[])
                  n474 = Not A Number/Path/Refnum?(number/path/refnum=w1289) -> (NaN/Path/Refnum?=w1288:bool[])
                  n475 = call "In_Range_check.vi"("±"=0.005, "%"=w1301, "Mode"=In_Range."% & ±", "Value"=w1292, "Setpoint"=w1293) -> ("In Range"=w1295:bool)  [unwired: 2 out]
                  n476 = call "In_Range_check.vi"("±"=0.005, "%"=w1298, "Mode"=In_Range."% & ±", "Value"=w1290, "Setpoint"=w1291) -> ("In Range"=w1296:bool)  [unwired: 2 out]
                  n477 = And(x=w1295, y=w1296) -> (x .and. y?=w1294:bool)
                }
                frame #1 {
                  n478 = case shown="False" w1315 {
                    tunnel: [0.0 w1317] -> w1314
                    tunnel: w1313 -> [_ w1322]
                    tunnel: w1312 -> [_ w1318]
                    tunnel: w1311 -> [_ w1321]
                    frame False {
                    }
                    frame True {
                      n479 = Or Array Elements(Boolean array=w1321) -> (logical OR=w1320:bool)
                      n480 = Add(x=w1322, y=w1318) -> (x+y=w1319:dbl)
                      n481 = Select(t=w1318, s=w1320, f=w1319) -> (s? t:f=w1317:dbl)
                    }
                  }
                }
              }
            }
          }
        }
        frame "AutoZero" {
          n482 = call "CPP-ZeroMonitor.vi"("Scan Period"=w1327, "Previous Scan Value"=w1323, "Present scan array"=w1328, "Value to Output"=w1326, "Ch Description"=w1329, "Ch names"=w1330) -> ("Scan comment"=w1325:string, "Output"=w1324:dbl)  [unwired: 1 in, 1 out]
        }
        frame "Average", "St Deviation" {
          n483 = call "Stats.vi"("Scan Period"=w1336, "Present scan array"=w1335, "Ch Description"=w1338, "Ch names"=w1337) -> ("String"=w1331:string, "Stat"=w1334:dbl)  [unwired: 3 in, 1 out]
          n484 = Empty String/Path?(string/path=w1331) -> (empty?=w1333:bool)
          n485 = case shown="False" w1333 {
            tunnel: [w1340 w1345] -> w1332
            tunnel: w1331 -> [w1341 w1345]
            frame False {
              n486 = global read "ADAM_Global.vi" "Scan Index"() -> (w1343:i32)
              n487 = Greater?(x=w1343, y=15) -> (0:w1342:bool)
              n488 = Select(t=w1341, s=w1342, f="") -> (s? t:f=w1340:string)
            }
            frame True {
            }
          }
        }
        frame "Coded" {
        }
        frame "Client Info" {
          n489 = global read "ADAM_Global.vi" "Client State Array"() -> (w1360:T13[])
          n490 = call "Split_Ch_name.vi"("Ch name"=w1354) -> ("Top level"=w1352:string, "Low level"=w1350:string)  [unwired: 1 out]
          n491 = Equal?(x="Status" ("Substring"), y=w1352) -> (x = y?=w1351:bool)
          n492 = Select(t=w1350, s=w1351, f="") -> (s? t:f=w1348:string)
          n493 = for {
            tunnel: w1360 -> [w1369] mode=indexing
            tunnel: [w1368] -> w1361 mode=indexing
            n494 = Unbundle By Name(w1369) -> ("Client Name"=w1368:string)
          }
          n495 = Search 1D Array(1D array=w1361, element=w1348) -> (index of element=w1356:i32)  [unwired: 1 out]
          n496 = Less Than 0?(x=w1356) -> (x < 0?=w1355:bool)
          n497 = Index Array(array=w1360, index=w1356) -> (element=w1359:T13)
          n498 = case shown="False" w1355 {
            tunnel: w1359 -> [w1364 _]
            tunnel: w1348 -> [w1363 w1366]
            tunnel: [w1362 w1365] -> w1358
            frame False {
              n499 = call "Get_Client_Status_string.vi"("Client State Cluster"=w1364, "Client Name"=w1363) -> ("Code Value"=w1362:dbl)  [unwired: 1 in]
            }
            frame True {
              w1365 = 7.0 ("Code Value")
              n500 = call "Remember_value.vi"("Mode"=Remember_value_mode."Read and Write", "Input Value"=w1365, "Ch name"=w1366) -> ()  [unwired: 1 out]
            }
          }
        }
        frame "Comparator" {
          n501 = call "Comparator.vi"("Previous Scan Value"=w1370, "Present scan array"=w1373, "Ch Description"=w1374, "Ch names"=w1375) -> ("String"=w1371:string, "Value"=w1372:dbl)  [unwired: 3 in, 1 out]
        }
        frame "mapCompare" {
          n502 = disable-structure shown="Disabled" {
            disable-tunnel: w1381 -> [w1387 _]
            disable-tunnel: w1380 -> [w1386 _]
            disable-tunnel: w1379 -> [w1385 _]
            disable-tunnel: [w1384 _] -> w1378
            disable-tunnel: [w1383 _] -> w1377
            disable-tunnel: w1376 -> [w1382 _]
            frame Disabled {
              n503 = call "MapCompare.vi"("Previous Scan Value"=w1382, "Present scan array"=w1385, "Ch Description"=w1386, "Ch names"=w1387) -> ("Scan comment"=w1384:string, "Output"=w1383:dbl)  [unwired: 3 in, 1 out]
            }
            frame Enabled {
            }
          }
        }
        frame "Equation" {
          n504 = call "CPP-Equation.vi"("Scan Period"=w1392, "Previous Scan Value"=w1388, "Present scan array"=w1393, "Value to Output"=w1391, "Ch Description"=w1394, "Ch names"=w1395) -> ("Scan comment"=w1390:string, "Output"=w1389:dbl)  [unwired: 1 in, 1 out]
        }
        frame "Hold Value" {
        }
        frame "Read Ch" {
          n505 = Unbundle By Name(w1401) -> ("String"=w1398:string)
          n506 = call "Read_value_of_earlier_Ch.vi"("Desired Ch to Read"=w1398, "Ch names"=w1402, "Present scan array"=w1403) -> ("Value"=w1399:dbl, "Scan comment"=w1400:string)  [unwired: 1 in]
        }
        frame "Read A" {
          n507 = Unbundle By Name(w1405) -> ("A"=w1404:dbl)
        }
        frame "ScanPacer" {
          # "Computes delay to use to achieve \"A\" ms scan period"
          n508 = call "ADAMPacer.vi"("Scan Period"=w1407, "Previous Scan Value"=w1408, "Ch Description"=w1411) -> ("Scan comment"=w1409:string, "slug(s)"=w1410:dbl)  [unwired: 4 in, 1 out]
        }
        frame "Count Down Timer" {
          n509 = Equal To 0?(x=w1413) -> (x = 0?=w1412:bool)
          n510 = case shown="False" w1412 {
            tunnel: w1416 -> [w1426 _]
            tunnel: [w1423 w1430] -> w1415
            tunnel: w1413 -> [w1424 w1430]
            frame False {
              n511 = Absolute Value(x=w1424) -> (abs(x)=w1425:dbl)
              n512 = Greater Than 0?(x=w1424) -> (x > 0?=w1419:bool)
              n513 = Subtract(x=w1425, y=w1426) -> (x-y=w1422:dbl)
              n514 = Less Than 0?(x=w1422) -> (x < 0?=w1417:bool)
              n515 = Select(t=0.0, s=w1417, f=w1422) -> (s? t:f=w1420:dbl)
              n516 = Or(x=w1417, y=w1419) -> (x .or. y?=w1418:bool)
              n517 = case shown="True" w1418 {
                tunnel: [w1427 w1429] -> w1423
                tunnel: w1420 -> [w1428 w1429]
                frame False {
                  n518 = Negate(x=w1428) -> (-x=w1427:dbl)
                }
                frame True {
                }
              }
            }
            frame True {
            }
          }
        }
        frame "Test" {
          n519 = Subtract(x=w1431, y=2969882881.0) -> (x-y=w1435:dbl)
          n520 = Multiply(x=w1435, y=0.0005) -> (x*y=w1432:dbl)
          n521 = Random Number (0-1)() -> (number: 0 to 1=w1433:dbl)
          n522 = Add(x=w1433, y=w1432) -> (x+y=w1438:dbl)
        }
        frame "Web Client" {
          w1447 = 7200.0  # 2 Hours in Seconds
          n523 = Concatenate Strings(w1456, ":Last read" ("Substring")) -> (w1454:string)
          n524 = call "Remember_value.vi"("Mode"=Remember_value_mode."Read only", "Ch name"=w1454) -> ("Output Value"=w1453:dbl)  [unwired: 1 in]
          n525 = Not A Number/Path/Refnum?(number/path/refnum=w1453) -> (NaN/Path/Refnum?=w1451:bool)
          n526 = Subtract(x=w1439, y=w1453) -> (x-y=w1459:dbl)
          n527 = Greater?(x=w1459, y=1800.0) -> (0:w1452:bool)
          n528 = Or(x=w1452, y=w1451) -> (x .or. y?=w1440:bool)
          n529 = case shown="True" w1440 {
            frame False {
            }
            frame True {
              n530 = global read "Constants_global.vi" "EnFlo SW Folder"() -> (w1462:path)
              n531 = Build Path(base path=w1462, name or relative path=path "ADAM Server/SoftwareChannels/Web_Client.vi") -> (appended path=w1461:path)
              n532 = Open VI Reference(vi path=w1461) -> (vi reference=w1466:refnum<vi>, error out=w1467:errorcluster)  [unwired: 1 in, 4 out]
              n533 = property class="VI"(reference=w1466, error in=w1467) -> (reference out=w1469:refnum<vi>, error out=w1470:errorcluster, "Front Panel Window:Open"=w1468:bool)
              n534 = case shown="False" w1468 {
                tunnel: w1469 -> [w1476 w1479]
                tunnel: w1470 -> [w1475 w1478]
                tunnel: [w1474 w1479] -> w1471
                tunnel: [w1473 w1478] -> w1472
                frame False {
                  n535 = property class="VI"(reference=w1476, error in=w1475, "Front Panel Window:Open"=TRUE) -> (reference out=w1474:refnum<vi>, error out=w1473:errorcluster)
                }
                frame True {
                }
              }
              n536 = invoke class="VI" method="Run VI"(reference=w1471, error in=w1472, "Wait until done"=FALSE, "Auto Dispose Ref"=TRUE) -> ()  [unwired: 1 in, 5 out]
            }
          }
          n537 = Concatenate Strings(w1456, ":value time" ("Substring")) -> (w1442:string)
          n538 = call "Remember_value.vi"("Mode"=Remember_value_mode."Read only", "Ch name"=w1456) -> ("Output Value"=w1460:dbl)  [unwired: 1 in]
          n539 = call "Remember_value.vi"("Mode"=Remember_value_mode."Read only", "Ch name"=w1442) -> ("Output Value"=w1446:dbl)  [unwired: 1 in]
          n540 = Subtract(x=w1439, y=w1446) -> (x-y=w1445:dbl)
          n541 = Greater?(x=w1445, y=w1447) -> (0:w1450:bool)
          n542 = case shown="True" w1450 {
            tunnel: w1445 -> [_ w1485]
            tunnel: 3600.0 ("y") -> [_ w1484]
            tunnel: ["" w1482] -> w1449
            frame False {
            }
            frame True {
              n543 = Divide(x=w1485, y=w1484) -> (x/y=w1481:dbl)
              n544 = Format Into String(format string="Value is %.0f hours old." ("Format String"), w1481) -> (resulting string=w1482:string)  [unwired: 2 in, 1 out]
            }
          }
        }
        frame "Set Motor RPM" {
          n545 = Unbundle By Name(w1499) -> ("Port Name"=w1498:string, "Ch."=w1493:i32)
          n546 = Unbundle By Name(w1492) -> ("A"=w1490:dbl, "B"=w1491:dbl, "D"=w1489:dbl)
          n547 = for {
            N: w1493 -> [_]
            tunnel: w1498 -> [w1519]
            tunnel: w1488 -> [w1514]
            tunnel: [w1517] -> w1497 mode=indexing
            tunnel: w1491 -> [w1513]
            tunnel: w1490 -> [w1512]
            tunnel: w1489 -> [w1507]
            tunnel: [w1505] -> w1487 mode=indexing
            i -> [w1516]
            n548 = Increment(x=w1516) -> (x+1=w1515:i32)
            n549 = case shown="2" w1515 {
              tunnel: w1514 -> [w1520 w1521]
              tunnel: [w1520 w1522] -> w1506
              tunnel: w1513 -> [_ w1526]
              tunnel: w1512 -> [_ w1524]
              frame Default {
              }
              frame 2 {
                n550 = Multiply(x=w1521, y=w1526) -> (x*y=w1525:dbl)
                n551 = Add(x=w1524, y=w1525) -> (x+y=w1523:dbl)
                n552 = Add(x=w1521, y=w1523) -> (x+y=w1522:dbl)
              }
            }
            n553 = Greater?(x=w1506, y=w1507) -> (0:w1509:bool)
            n554 = Select(t=w1507, s=w1509, f=w1506) -> (s? t:f=w1511:dbl)
            n555 = Not A Number/Path/Refnum?(number/path/refnum=w1511) -> (NaN/Path/Refnum?=w1510:bool)
            n556 = Select(t=0.0, s=w1510, f=w1511) -> (s? t:f=w1505:dbl)
            n557 = call "Set motor RPM.vi"("RPM (/min)"=w1505, "Drive address"=w1515, "COM port"=w1519) -> ("Modbus error cluster"=w1518:T15)  [unwired: 1 in, 1 out]
            n558 = Unbundle By Name(w1518) -> ("Comms error"=w1517:errorcluster)
          }
          n559 = Index Array(array=w1487) -> (element=w1486:dbl)  [unwired: 1 in]
          n560 = Merge Errors(w1497) -> (w1496:errorcluster)
          n561 = case shown="Error .." w1496 {
            selector: w1496 -> [_ w1504]
            tunnel: ["" w1503] -> w1495
            tunnel: w1486 -> [w1500 _]
            tunnel: [w1500 nan ("Value to Output")] -> w1494
            frame No Error {
            }
            frame Error {
              n562 = Unbundle By Name(w1504) -> ("source"=w1503:string)
            }
          }
        }
        frame "Read Motor Info" {
          n563 = Unbundle By Name(w1538) -> ("Port Name"=w1535:string, "Ch."=w1530:i32)
          n564 = for {
            N: w1530 -> [_]
            tunnel: w1535 -> [w1546]
            tunnel: [w1544] -> w1534 mode=indexing
            tunnel: [w1543] -> w1533 mode=indexing
            tunnel: [w1542] -> w1532 mode=indexing
            tunnel: [w1540] -> w1529 mode=indexing
            tunnel: [w1539] -> w1527 mode=indexing
            i -> [w1541]
            n565 = Increment(x=w1541) -> (x+1=w1539:i32)
            n566 = call "Get further extended drive and motor status.vi"("COM port"=w1546, "Drive address"=w1539) -> ("Modbus error cluster"=w1545:T15, "Extended drive status"=w1544:T17, "Motor data"=w1543:T18, "Further motor and drive data"=w1542:T19)  [unwired: 9 in, 1 out]
            n567 = Unbundle By Name(w1545) -> ("Comms error"=w1540:errorcluster)
          }
          n568 = Merge Errors(w1529) -> (w1528:errorcluster)
          n569 = case shown="Error .." w1528 {
            selector: w1528 -> [_ w1589]
            tunnel: ["" w1588] -> w1537
            tunnel: [w1557 nan ("Value to Output")] -> w1536
            tunnel: w1534 -> [w1558 _]
            tunnel: w1533 -> [w1556 _]
            tunnel: w1532 -> [w1555 _]
            tunnel: w1531 -> [w1554 _]
            tunnel: w1527 -> [w1547 _]
            frame No Error {
              n570 = for {
                tunnel: w1558 -> [w1579] mode=indexing
                tunnel: w1556 -> [w1570] mode=indexing
                tunnel: w1555 -> [w1569] mode=indexing
                tunnel: w1554 -> [w1565]
                tunnel: [w1563] -> w1551 mode=concatenating
                tunnel: [w1561] -> w1550 mode=indexing
                tunnel: w1547 -> [w1562] mode=indexing
                n571 = Unbundle By Name(w1570) -> ("Motor RPM (/min)"=w1573:dbl, "Motor current (A)"=w1575:dbl, "Motor power (kW)"=w1574:dbl, "Motor torque (%)"=w1576:dbl)
                n572 = Unbundle By Name(w1569) -> ("Drive internal temperature (°C)"=w1578:dbl)
                n573 = Match Pattern(string=w1565, regular expression=":") -> (before substring=w1564:string)  [unwired: 1 in, 3 out]
                n574 = Build Array(w1573, w1575, w1574, w1576, w1578) -> (w1577:dbl[])
                n575 = Format Into String(format string="%s:Motor %d:", w1564, w1562) -> (resulting string=w1572:string)  [unwired: 2 in, 1 out]
                n576 = Unbundle By Name(w1579) -> ("Standby"=w1561:bool)
                n577 = for {
                  tunnel: w1572 -> [w1586]
                  tunnel: string[] ["RPM", "Current (A)", "Power (kW)", "Torque (%)", "Drive Temp"] -> [w1585] mode=indexing
                  tunnel: T11 {"Channel Name"="", "New Value"=0.0, "!Auto_Off"=FALSE} ("Update Scan Value Cluster") -> [w1584]
                  tunnel: w1577 -> [w1581] mode=indexing
                  tunnel: [w1580] -> w1563 mode=indexing
                  n578 = Concatenate Strings(w1586, w1585) -> (w1583:string)
                  n579 = Bundle By Name(cluster=w1584, "Channel Name"=w1583, "New Value"=w1581, "!Auto_Off"=TRUE) -> (w1580:T11)
                }
              }
              n580 = And Array Elements(Boolean array=w1550) -> (logical AND=w1549:bool)
              n581 = Select(t=1.0, s=w1549, f=0.0) -> (s? t:f=w1557:dbl)
              n582 = call "Update_Current_Value_server.vi"("Mode"=T10."Append to Global", "Client HD name"="ADAM Server", "Update array in"=w1551) -> ()  [unwired: 1 out]
            }
            frame Error {
              n583 = Unbundle By Name(w1589) -> ("source"=w1588:string)
            }
          }
        }
        frame "Run VI Named:" {
          n584 = call "DoRunVInamed.vi"("Scan Period"=w1593, "Previous Scan Value"=w1594, "Present scan array"=w1595, "Value to Output"=w1596, "Ch Description"=w1590, "Ch names"=w1597) -> ("Scan comment"=w1591:string, "Output"=w1592:dbl)  [unwired: 1 in, 1 out]
        }
        frame "Oops", Default {
        }
      }
    }
    frame #2 {
      n585 = call <vilib>:"High Resolution Relative Seconds.vi"() -> ("relative seconds"=w1602:dbl)
      n586 = Subtract(x=w1602, y=w1601) -> (x-y=w1600:dbl)
    }
  }
  "Output" <- w6
  "Scan comment" <- w7
  "execTime" <- w1
